vi "Retrieve and visualize_noDVR.vi"(11 "Field/Temperature":i32(slide) min=0 max=36 step=1) -> (1 "slowest":dbl format="%#_6p")   [LabVIEW 2020, in "Retrieve and Visualize.lvclass"]
uses:
  Retrieve and Visualize.lvclass
  typedefs/IV Setup--Cluster.ctl
  typedefs/Choose Intensity Data--enum.ctl
  <userlib>/LevyLab/LV-Data/LV-Data/Typedefs/File Type--enum.ctl
  typedefs/Choose XY Data--enum.ctl
  <userlib>/LevyLab/Graph Utilities/graph_utilities.lvclass
  <userlib>/LevyLab/Instrument Framework/SMOs/Configuration/Configuration.lvclass
  typedefs/INI--Cluster.ctl
  <vilib>/Utility/sysdir.llb/System Directory Type.ctl
  <userlib>/LevyLab/Graph Utilities/graph_utilities.lvclass/graph_utilities.ctl
  Retrieve and Visualize.lvclass/Retrieve and Visualize.ctl
  <userlib>/LevyLab/XY Utilities/subVIs/Subset (multiple).vi
  <userlib>/LevyLab/XY Utilities/subVIs/Sort (multiple).vi
  <userlib>/LevyLab/XY Utilities/subVIs/Decimate (multiple).vi
  <userlib>/LevyLab/XY Utilities/subVIs/Savitsky Golay Filter (multiple).vi
  <userlib>/LevyLab/XY Utilities/subVIs/Difference Quotient (multiple).vi
  <vilib>/Analysis/baseanly.llb/A x B.vi
  <vilib>/Analysis/baseanly.llb/A x Vector.vi
  <userlib>/LevyLab/XY Utilities/subVIs/Subset (single).vi
  <userlib>/LevyLab/XY Utilities/subVIs/Sort (single).vi
  <userlib>/LevyLab/XY Utilities/subVIs/Decimate (single).vi
  <userlib>/LevyLab/XY Utilities/subVIs/Savitsky Golay Filter (single).vi
  <userlib>/LevyLab/XY Utilities/subVIs/Difference Quotient (single).vi
  <vilib>/Analysis/2dsp.llb/Decimate (single shot).vi
  <vilib>/Analysis/2dsp.llb/Decimate (single shot, DBL).vi
  <vilib>/Analysis/3filter.llb/Savitzky-Golay Filter.vi
  <vilib>/Analysis/3filter.llb/Savitzky-Golay Filter (DBL).vi
  <userlib>/LevyLab/XY Utilities/Private/X Units.vi
  <userlib>/LevyLab/XY Utilities/Swap X and Y.vi
  <userlib>/LevyLab/XY Utilities/subVIs/Swap X and Y (single).vi
  <userlib>/LevyLab/XY Utilities/Private/DQ subVI.vi
  <userlib>/LevyLab/XY Utilities/Reverse.vi
  <userlib>/LevyLab/XY Utilities/subVIs/Reverse (single).vi
  <userlib>/LevyLab/XY Utilities/Divide.vi
  <userlib>/LevyLab/XY Utilities/subVIs/Divide float (single).vi
  <userlib>/LevyLab/XY Utilities/Add.vi
  <userlib>/LevyLab/XY Utilities/subVIs/Add XY (single).vi
  <userlib>/LevyLab/XY Utilities/Private/X Array Range to Index.vi
  <userlib>/LevyLab/Graph Utilities/Intensity Graph/Set Intensity Graph Cursor.vi
  <userlib>/LevyLab/Graph Utilities/Intensity Graph/Get Intensity Graph X Scale.vi
  <userlib>/LevyLab/Graph Utilities/Intensity Graph/Get Intensity Graph Value.vi
  <userlib>/LevyLab/Graph Utilities/Intensity Graph/Get Intensity Graph Y Scale.vi
  <userlib>/LevyLab/Graph Utilities/subVIs/Step Average.vi
  <userlib>/LevyLab/Graph Utilities/subVIs/Normalized Gaussian.vi
  <userlib>/LevyLab/Graph Utilities/XY Graph/Set XY Graph Value (array).vi
  <userlib>/LevyLab/Graph Utilities/Intensity Graph/Get Intensity Graph Y Label.vi
  <userlib>/LevyLab/Graph Utilities/XY Graph/Set XY Graph X Label.vi
  <userlib>/LevyLab/Graph Utilities/Intensity Graph/Get Intensity Graph Z Label.vi
  <userlib>/LevyLab/Graph Utilities/XY Graph/Set XY Graph Y Label.vi
  <userlib>/LevyLab/Graph Utilities/Intensity Graph/Get Intensity Graph X Label.vi
  <userlib>/_OpenG.lib/file/file.llb/File Exists - Scalar__ogtk.vi
  <userlib>/_OpenG.lib/array/array.llb/Sort Array__ogtk.vi
  <userlib>/_OpenG.lib/array/array.llb/Sort 1D Array (DBL)__ogtk.vi
  <userlib>/_OpenG.lib/array/array.llb/Reorder Array2__ogtk.vi
  <userlib>/_OpenG.lib/array/array.llb/Reorder 1D Array2 (DBL)__ogtk.vi
  <vilib>/Analysis/NI_AAL_SigProc.lvlib
  <userlib>/LevyLab/XY Utilities/xy_utilities.lvlib
  <userlib>/LevyLab/XY Utilities/subVIs/Interpolate (single).vi
  <userlib>/LevyLab/XY Utilities/Typedefs/Interpolation Configuration--cluster.ctl
  <userlib>/LevyLab/LV-Data/LV-Data.ITX/LV-Data.ITX.lvclass
  <userlib>/LevyLab/LV-Data/LV-Data/LV-Data.lvclass
panel:
  out "Status":string
  in  "Tab Control 2":enum32{"Sweep Control", "Visualize"}(tab)=enum."Visualize"
  out "Cursor Graph":cluster{dbl[], dbl[]}(graph)={[0.099856, 0.1204, 0.1401, 0.1599, 0.1798, 0.1998, 0.2198, 0.2398, 0.2598, 0.2798, 0.2998, 0.3199, 0.3398, 0.3598, 0.3798, 0.4, 0.4196, 0.4398, 0.4598, 0.4796, 0.5, 0.52, 0.5399, 0.5597, 0.5799, 0.5997, 0.62, 0.6398, 0.6601, 0.68, 0.6997, 0.7198, 0.7399, 0.7598, 0.78, 0.8002, 0.8201, 0.8401, 0.8597, 0.8797, 0.9, 0.9198, 0.9399, 0.96, 0.9798, 0.9802, 1.0002, 1.0202, 1.0404, 1.0602, 1.0807], [0.999930859375, 0.999930859375, 0.999930859375, 0.999930859375, 0.999930859375, 0.999930859375, 0.999930859375, 0.999930859375, 0.999930859375, 0.999930859375, 0.999930859375, 0.999930859375, 0.999930859375, 0.999930859375, 0.999930859375, 0.999930859375, 0.999930859375, 0.999930859375, 0.999930859375, 0.999930859375, 0.999930859375, 0.999930859375, 0.999930859375, 0.999930859375, 0.999930859375, 0.999930859375, 0.999930859375, 0.999930859375, 0.999930859375, 0.999930859375, 0.999930859375, 0.999930859375, 0.999930859375, 0.999930859375, 0.999930859375, 0.999930859375, 0.999930859375, 0.999930859375, 0.999930859375, 0.999930859375, 0.999930859375, 0.999930859375, 0.999930859375, 0.999930859375, 0.999930859375, 0.999930859375, 0.999930859375, 0.999930859375, 0.999930859375, 0.999930859375, 0.999930859375]}
  out "Fast":dbl=-2.603786046511628
  out "Slow":dbl=0.023622047244094446
  in  "decimating factor (1)":i32=1
  in  "averaging":bool
  in  "S-G side points (2T)":i32=10
  in  "S-G side points (4T)":i32=10
  in  "Subset Slider (%) A":cluster{dbl, dbl}(slide)={100.0, 0.0} scale=0.0..100.0 scale format="%#_6f"
  in  "Window [h]":dbl=10.0 min=2.0
  in  "Transconductance [h]":dbl=10.0 min=2.0
  in  "Visualize Button":bool
  in  "Open DAT Path":path=path "G:/.shortcut-targets-by-id/0B8-gGFa6hkR4XzJJMDlqZXVKRk0/ansom/Data/PPMS 3/SA40511C.20250205/000-processed/10-IV1TWire1nd2_Tsweep.000002.dat"
  in  "Macro: Visualize":string="Data Visualize: Read DAT File\nData Visualize: Initialize Graphs\nData Visualize: Initialize Cursor Graph\nData Visualize: Subset\nData Visualize: Testing\nData Visualize: SG Filter\nData Visualize: Calculate Derivative 2T\nData Visualize: Calculate Derivative 4T\nData Visualize: IV 4T IV 2T\n//Data Visualize: Calculate Transconductance\nData Visualize: Calculate Indices\nGraph: Initialize\nGraph: Set Y\nGraph: Set Labels\n//Data Visualize: Calculate Indices\n//Data Visualize: Choose Data 1\n//Data Visualize: Choose Data 2\n//Graph: Linecuts\n//UI: Choose Tab >> Intensity Graphs\nUI: Cursor Set >> Idle"
  in  "OK":bool
  in  "Tab Control":T1(tab)=enum."Intensity Graphs"
  out "Comments":string="      #Vslow/#Vfast/# of IV curves/BT offset/#discarded IV curves/Manual offset:\n /1/51/1/0/0/0    \n#of fields: 1    \nField period 1 \nDecimate point 1.000000 \nScan names \nT (K)\nB (T)\nappliedField \n Device: \r  Device Name: SA40511C.20250205\r  Computer: PPMS3DAQ\r  User: Ranjani\r  Instrument: PPMS 3\r  Description: |\r    LAO/KTO 3wire Nernst\r\rExperiment: \r  Time: 2025-02-08T22:02:51\r  Description: |\r    T = 100mK to 980mK, 20mK step,10K/min \r    Wait(temperature)\r    B= 1T\r    \r    I1 and 2+= 0 to -50m to 50m to 0V, 30s\r    wait, 2s\r    I+/- = 2/5\r    V+/- = 1/26\r    I2+/- = 3/4\r    Wire 3\r    I3+/- = 0 mV\r\rSweep: \r- Loop1: [Temperature, 1.080000]\r- Loop2: [OFF, -14.000000]\r- Loop3: [OFF, 0.000000]\r- Loop4: [OFF, 0.000000]\r\rWiring: \r- Electrode 1: Lockin 1, V1+\r- Electrode 2: Lockin 2, I+\r- Electrode 3: Lockin 3, I2+\r- Electrode 4: Lockin 4, I2-\r- Electrode 5: Lockin 5, I-\r- Electrode 26: Lockin 6, V1-\r- Electrode 27: Lockin 7, I3+\r- Electrode 28: Lockin 8, I3+\r\rLockin: \r  AO: \r  - AO 1: amp = 0.000 mV, DC = 0.000 mV, f = 13.00 Hz, phi = 0.00°, Sine\r  - AO 2: amp = 0.000 mV, DC = 0.001 mV, f = 13.00 Hz, phi = 0.00°, Sine\r  - AO 3: amp = 0.000 mV, DC = 0.001 mV, f = 13.00 Hz, phi = 0.00°, Sine\r  - AO 4: amp = 0.000 mV, DC = 0.000 mV, f = 13.00 Hz, phi = 0.00°, Sine\r  - AO 5: amp = 0.000 mV, DC = 0.000 mV, f = 13.00 Hz, phi = 0.00°, Sine\r  - AO 6: amp = 0.000 mV, DC = 0.000 mV, f = 13.00 Hz, phi = 0.00°, Sine\r  - AO 7: amp = 0.000 mV, DC = 0.000 mV, f = 13.00 Hz, phi = 0.00°, Sine\r  - AO 8: amp = 0.000 mV, DC = 0.000 mV, f = 13.00 Hz, phi = 0.00°, Sine\r  REF: \r  - Lockin 1: f = 13.00 Hz, phi = 0.00°, TC = 0.10 s, order = 2 \r  - Lockin 2: f = 26.00 Hz, phi = 0.00°, TC = 0.10 s, order = 2 \r  Sampling: \r  - Fs: 13000.000000\r  - N: 1000\r"
  in  "index":T2={"I-(A)"="AO2", "I+(A)"="AI5", "V4T+"="AI1", "V4T-"="AI6", "UG"="AO1", "DG"="AO1", "LG"="AO6", "B"="Magnet", "Temperature"="Temperature", "Vfast"="Temperature", "Vslow"="Magnet"}
  in  "Check Files Button":bool
  in  "Generate Button":bool
  in  "Additional comments":string
  in  "Field Period":i32=1
  in  "# of fields/Temperatures":i32=1
  in  "Path":path=path "G:/.shortcut-targets-by-id/0B8-gGFa6hkR4XzJJMDlqZXVKRk0/ansom/Data/PPMS 3/SA40511C.20250205/10-IV1TWire1nd2_Tsweep"
  in  "DAT folder":path=path "G:/.shortcut-targets-by-id/0B8-gGFa6hkR4XzJJMDlqZXVKRk0/ansom/Data/PPMS 3/SA40511C.20250205/000-processed"
  in  "IV setup":T3={"# Vslow"=1, "# Vfast"=51, "#IV Curves at each gate"=1, "B/T offset"=0, "Discard first # curves"=0, "Manual offset"=0}
  in  "Scan names":string[](array[string])=["T (K)", "B (T)", "appliedField"]
  in  "Portion of data (%)":cluster{dbl, dbl}(slide)={100.0, 0.0} scale=0.0..100.0
  in  "Decimate point":dbl=1.0 format="%#_1f"
  in  "Extract paramaters from comments?":bool
  in  "T/B third axis":bool
  in  "File Type":T4=enum."TDMS"
  in  "Export ITX Path":path
  in  "Export ITX":bool
  in  "Export What?":T5(ring)
  in  "Export ITX Name":string
  out "IV 4T":cluster{dbl[], dbl[]}[](graph)
  out "dI/dV (G)":cluster{dbl[], dbl[]}[](graph)
  out "dI/dV (G) 2T":cluster{dbl[], dbl[]}[](graph)
  out "IV 2T":cluster{dbl[], dbl[]}[](graph)
  out "dV/dI (R)":cluster{dbl[], dbl[]}[](graph)
  out "dV/dI (R) 2T":cluster{dbl[], dbl[]}[](graph)
  in  "XY Data":T6
  in  "fake point 1":dbl format="%#_6p"
  in  "Log scale? 1":bool
  in  "e^2/h? 1":bool
  in  "e^2/h? 2":bool
  in  "Log scale? 2":bool
  in  "fake point 2":dbl=-2.0 format="%#_6p"
  in  "Intensity 1":T7=enum."R-4T"
  out "Intensity Graph 1":dbl[][](graph)
  out "Intensity Graph 2":dbl[][](graph)
  out "H Cut 1":cluster{dbl[], dbl[]}[](graph)
  out "V Cut 1":cluster{dbl[], dbl[]}[](graph)=[{[0.099856, 0.11947288, 0.13908976, 0.15870664, 0.17832352, 0.19794040000000002, 0.21755728, 0.23717416, 0.25679103999999997, 0.27640792000000003, 0.2960248, 0.31564168000000004, 0.33525856, 0.35487544, 0.37449232, 0.3941092, 0.41372608, 0.43334296, 0.45295984, 0.47257672, 0.4921936, 0.5118104800000001, 0.53142736, 0.55104424, 0.57066112, 0.590278, 0.6098948799999999, 0.62951176, 0.64912864, 0.6687455200000001, 0.6883623999999999, 0.70797928, 0.72759616, 0.7472130399999999, 0.7668299199999999, 0.7864468, 0.8060636800000001, 0.8256805599999999, 0.84529744, 0.86491432, 0.8845312000000001, 0.9041480799999999, 0.92376496, 0.94338184, 0.9629987200000001, 0.9826155999999999, 1.00223248, 1.02184936, 1.0414662399999999, 1.06108312, 1.0807], [nan, nan, nan, nan, nan, nan, nan, nan, nan, nan, nan, nan, nan, nan, nan, nan, nan, nan, nan, nan, nan, nan, nan, nan, nan, nan, nan, nan, nan, nan, nan, nan, nan, nan, nan, nan, nan, nan, nan, nan, nan, nan, nan, nan, nan, nan, nan, nan, nan, nan, nan]}]
  out "H Cut 2":cluster{dbl[], dbl[]}[](graph)
  out "V Cut 2":cluster{dbl[], dbl[]}[](graph)=[{[0.099856, 0.11947288, 0.13908976, 0.15870664, 0.17832352, 0.19794040000000002, 0.21755728, 0.23717416, 0.25679103999999997, 0.27640792000000003, 0.2960248, 0.31564168000000004, 0.33525856, 0.35487544, 0.37449232, 0.3941092, 0.41372608, 0.43334296, 0.45295984, 0.47257672, 0.4921936, 0.5118104800000001, 0.53142736, 0.55104424, 0.57066112, 0.590278, 0.6098948799999999, 0.62951176, 0.64912864, 0.6687455200000001, 0.6883623999999999, 0.70797928, 0.72759616, 0.7472130399999999, 0.7668299199999999, 0.7864468, 0.8060636800000001, 0.8256805599999999, 0.84529744, 0.86491432, 0.8845312000000001, 0.9041480799999999, 0.92376496, 0.94338184, 0.9629987200000001, 0.9826155999999999, 1.00223248, 1.02184936, 1.0414662399999999, 1.06108312, 1.0807], [3.3762685773770134e-05, 2.3916778489875587e-05, 2.654588549110859e-05, 3.7526761290691605e-05, 3.2301327892542505e-05, 2.6454434035762424e-05, 2.652299633224866e-05, 3.230184057865135e-05, 1.959244546016357e-05, 2.584103725701611e-05, 3.445648987553342e-05, 1.7963722001670446e-05, 1.4959654834668283e-05, 2.488740425029002e-05, 2.6029819241313776e-05, 2.0114406725304238e-05, 2.1938239917722983e-05, 2.3924326114769558e-05, 1.688456387309341e-05, 1.2689595493509836e-05, 2.1639531028779784e-05, 1.0262319510907414e-05, -2.2562712513605623e-06, 6.229663764846753e-06, 6.290560504043035e-06, -4.464216464504397e-06, -9.063974731389205e-06, 4.423251858920318e-06, -9.326548951846347e-06, -1.0215397278681526e-05, -9.304831257511187e-06, -8.915859738611292e-06, -1.9912084696571762e-05, -9.449798911587456e-06, -1.145229397349045e-05, -1.7712755942352026e-05, -2.02944113979962e-05, -1.313296945631493e-05, -2.420582028533799e-05, -2.348366665214838e-05, -1.8166676626836458e-05, -2.5173787476635757e-05, -3.2642280402476225e-05, -1.8777899023935893e-05, -2.788070158268089e-05, -7.192029457748351e-06, -1.8816023944703815e-05, -1.6190991731435217e-05, -1.1918852338953221e-05, -1.8801482914666336e-05, -2.1966004211086435e-05]}]
  in  "Intensity 2":T7
  in  "X Offset 1":dbl format="%#_6p"
  in  "X Offset 2":dbl format="%#_6p"
  out "x3D Graph 11":dbl[][](graph)
  out "x3D Graph 10":dbl[][](graph)
  out "x3D Graph 9":dbl[][](graph)
  out "x3D Transconductance 2":dbl[][](graph)
  in  "Intensity 3D":T7=enum."G-4T"
  out "bottom loop":dbl[](graph)
  out "xalpha top loop":dbl[](graph)
  out "xalpha Top loop Intensity Graph":dbl[][](graph)
  out "xalpha Vsd vs Vsg":cluster{dbl[], dbl[]}(graph)
  in  "xalpha threshold 2":dbl format="%0.2f"
  in  "xalpha width 2":i32=3 min=3
  out "xalpha Y line cut 9":cluster{dbl[], dbl[]}[](graph)
  out "xalpha Vsg?":dbl[](array[numeric])
  out "xalpha vertical peak diff":dbl[](array[numeric])
  in  "xalpha threshold":dbl format="%0.2f"
  in  "xalpha width":i32=3 min=3
  in  "xalpha derivative bin size":dbl=10.0
  in  "Diff Interval":dbl=12.0
  in  "derivative bin size 2":dbl
  in  "derivative bin size 1":dbl
  in  "SG Filter?":bool=TRUE
  # "Input"
  # "Process Parameters"
  # "obsolete?"
  # "Vfast"
  # "Vslow"
  # "Vslowest"
  # "Output"
  # "#todo: add button to automatically populate output and filename fields"
  # "Used??"
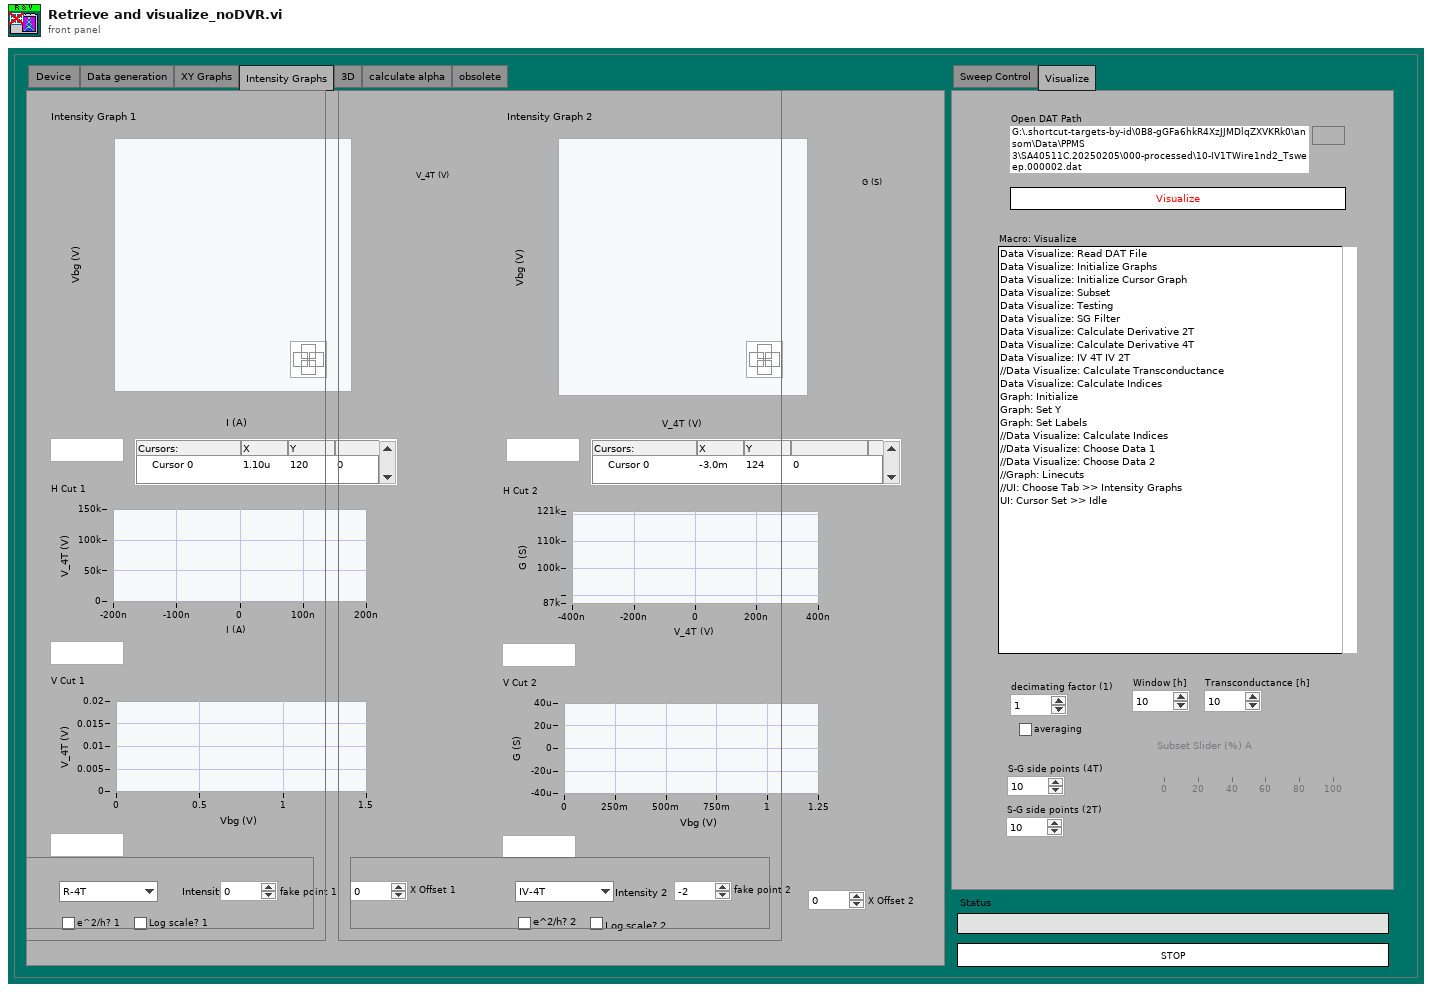
[diagram p1: front panel]
types:
  T1 = enum32{"Device ", "Data generation", "XY Graphs", "Intensity Graphs", "3D", "calculate alpha", "obsolete"}
  T2 = cluster{"I-(A)":string, "I+(A)":string, "V4T+":string, "V4T-":string, "UG":string, "DG":string, "LG":string, "B":string, "Temperature":string, "Vfast":string, "Vslow":string}
  T3 = typedef "Retrieve and Visualize.lvclass/IV Setup--Cluster.ctl" = cluster{"# Vslow":i32, "# Vfast":i32, "#IV Curves at each gate":i32, "B/T offset":i32, "Discard first # curves":i32, "Manual offset":i32}
  T4 = typedef "LV-Data.lvclass/File Type--enum.ctl" = enum16{"DAT", "ITX", "TDMS", "VI"}
  T5 = enum16{"Intensity 1", "H Cut 1", "V Cut 1", "Intensity 2", "H Cut 2", "V Cut 2"}
  T6 = typedef "Retrieve and Visualize.lvclass/Choose XY Data--enum.ctl" = enum16{"Vary Vfast", "Vary Vslow", "Vary Fields"}
  T7 = typedef "Retrieve and Visualize.lvclass/Choose Intensity Data--enum.ctl" = enum16{"IV-4T", "IV-2T", "R-4T", "G-4T", "R-2T", "G-2T", "dGdVsg-4T", "dGdVsg-2T"}
  T8 = enum32{"Device ", "Data generation", "Vary Vfast", "Vary Vslow", "Vary Fields", "Intensity Graphs", "3D (disabled)", "calculate alpha (disabled)"}
  T9 = cluster{"IV-4T":refnum<data-value>, "G-2T":refnum<data-value>, "R-2T":refnum<data-value>, "G-4T":refnum<data-value>, "R-4T":refnum<data-value>, "IV-2T":refnum<data-value>, "Vfast":dbl[][], "Vslow":dbl[], "Vslowest":dbl[], "Scan Names":string[]}
  T10 = typedef "xy_utilities.lvlib/Interpolation Configuration--cluster.ctl" = cluster{"X Low":dbl, "X High":dbl, "X Step":dbl, "Fake Point":dbl}
  T11 = typedef "LVOffsetAndMultiplierTypeDef.ctl" = cluster{"Offset":dbl, "Multiplier":dbl}
  T12 = enum32{"Invalid", "Standard", "Closed", "Hidden", "Minimized", "Maximized"}
  T13 = enum32{"invalid app kind", "Development System", "Run Time System", "Student Edition", "Embedded LabVIEW", "Evaluation", "Custom"}
  T14 = typedef "Retrieve and Visualize.lvclass/INI--Cluster.ctl" = cluster{"Open DAT Path":path, "Export ITX Path":path, "Export ITX Name":string, "Intensity 1":T7, "X Offset 1":dbl, "derivative bin size 1":dbl, "e^2/h? 1":bool, "Log scale? 1":bool, "fake point 1":dbl, "Intensity 2":T7, "X Offset 2":dbl, "derivative bin size 2":dbl, "e^2/h? 2":bool, "Log scale? 2":bool, "fake point 2":dbl}
  T15 = cluster{"Core":cluster{"Current VI Reference":refnum<vi>, "Close Panel on Exit?":bool}, "R&V":refnum<class "Retrieve and Visualize.lvclass">, "Configuration":refnum<class "Configuration.lvclass">, "INI":T14, "3D":cluster{"IV-4T":cluster{dbl[], dbl[]}[][][], "IV-2T":cluster{dbl[], dbl[]}[][][], "G-4T":cluster{dbl[], dbl[]}[][][], "R-4T":cluster{dbl[], dbl[]}[][][], "G-2T":cluster{dbl[], dbl[]}[][][], "R-2T":cluster{dbl[], dbl[]}[][][], "dG-4T":cluster{dbl[], dbl[]}[][][], "Differential Mode":cluster{dbl[], dbl[]}[][][], "Common Mode":cluster{dbl[], dbl[]}[][][]}, "Graph":cluster{"Intensity 1":refnum<class "graph_utilities.lvclass">, "V 1":refnum<class "graph_utilities.lvclass">, "H 1":refnum<class "graph_utilities.lvclass">, "Intensity 2":refnum<class "graph_utilities.lvclass">, "V 2":refnum<class "graph_utilities.lvclass">, "H 2":refnum<class "graph_utilities.lvclass">}, "Vfast":dbl[][], "Vslow":dbl[], "Vslowest":dbl[], "Scan Names":string[], "Vfast Slice":dbl[], "Vslow Slice":dbl[], "Page":i32, "Row":i32, "Column":i32, "Row []":i32[], "Column []":i32[], "V2T":dbl[]}
  T16 = cluster{"Intensity 1":refnum<class "graph_utilities.lvclass">, "V 1":refnum<class "graph_utilities.lvclass">, "H 1":refnum<class "graph_utilities.lvclass">, "Intensity 2":refnum<class "graph_utilities.lvclass">, "V 2":refnum<class "graph_utilities.lvclass">, "H 2":refnum<class "graph_utilities.lvclass">}
  T17 = cluster{"IV-4T":cluster{dbl[], dbl[]}[][][], "IV-2T":cluster{dbl[], dbl[]}[][][], "G-4T":cluster{dbl[], dbl[]}[][][], "R-4T":cluster{dbl[], dbl[]}[][][], "G-2T":cluster{dbl[], dbl[]}[][][], "R-2T":cluster{dbl[], dbl[]}[][][], "dG-4T":cluster{dbl[], dbl[]}[][][], "Differential Mode":cluster{dbl[], dbl[]}[][][], "Common Mode":cluster{dbl[], dbl[]}[][][]}
  T18 = cluster{"Current VI Reference":refnum<vi>, "Close Panel on Exit?":bool}
  T19 = typedef "System Directory Type.ctl" = i32
  T20 = typedef "LVPointDoubleTypeDef.ctl" = cluster{"X":dbl, "Y":dbl}
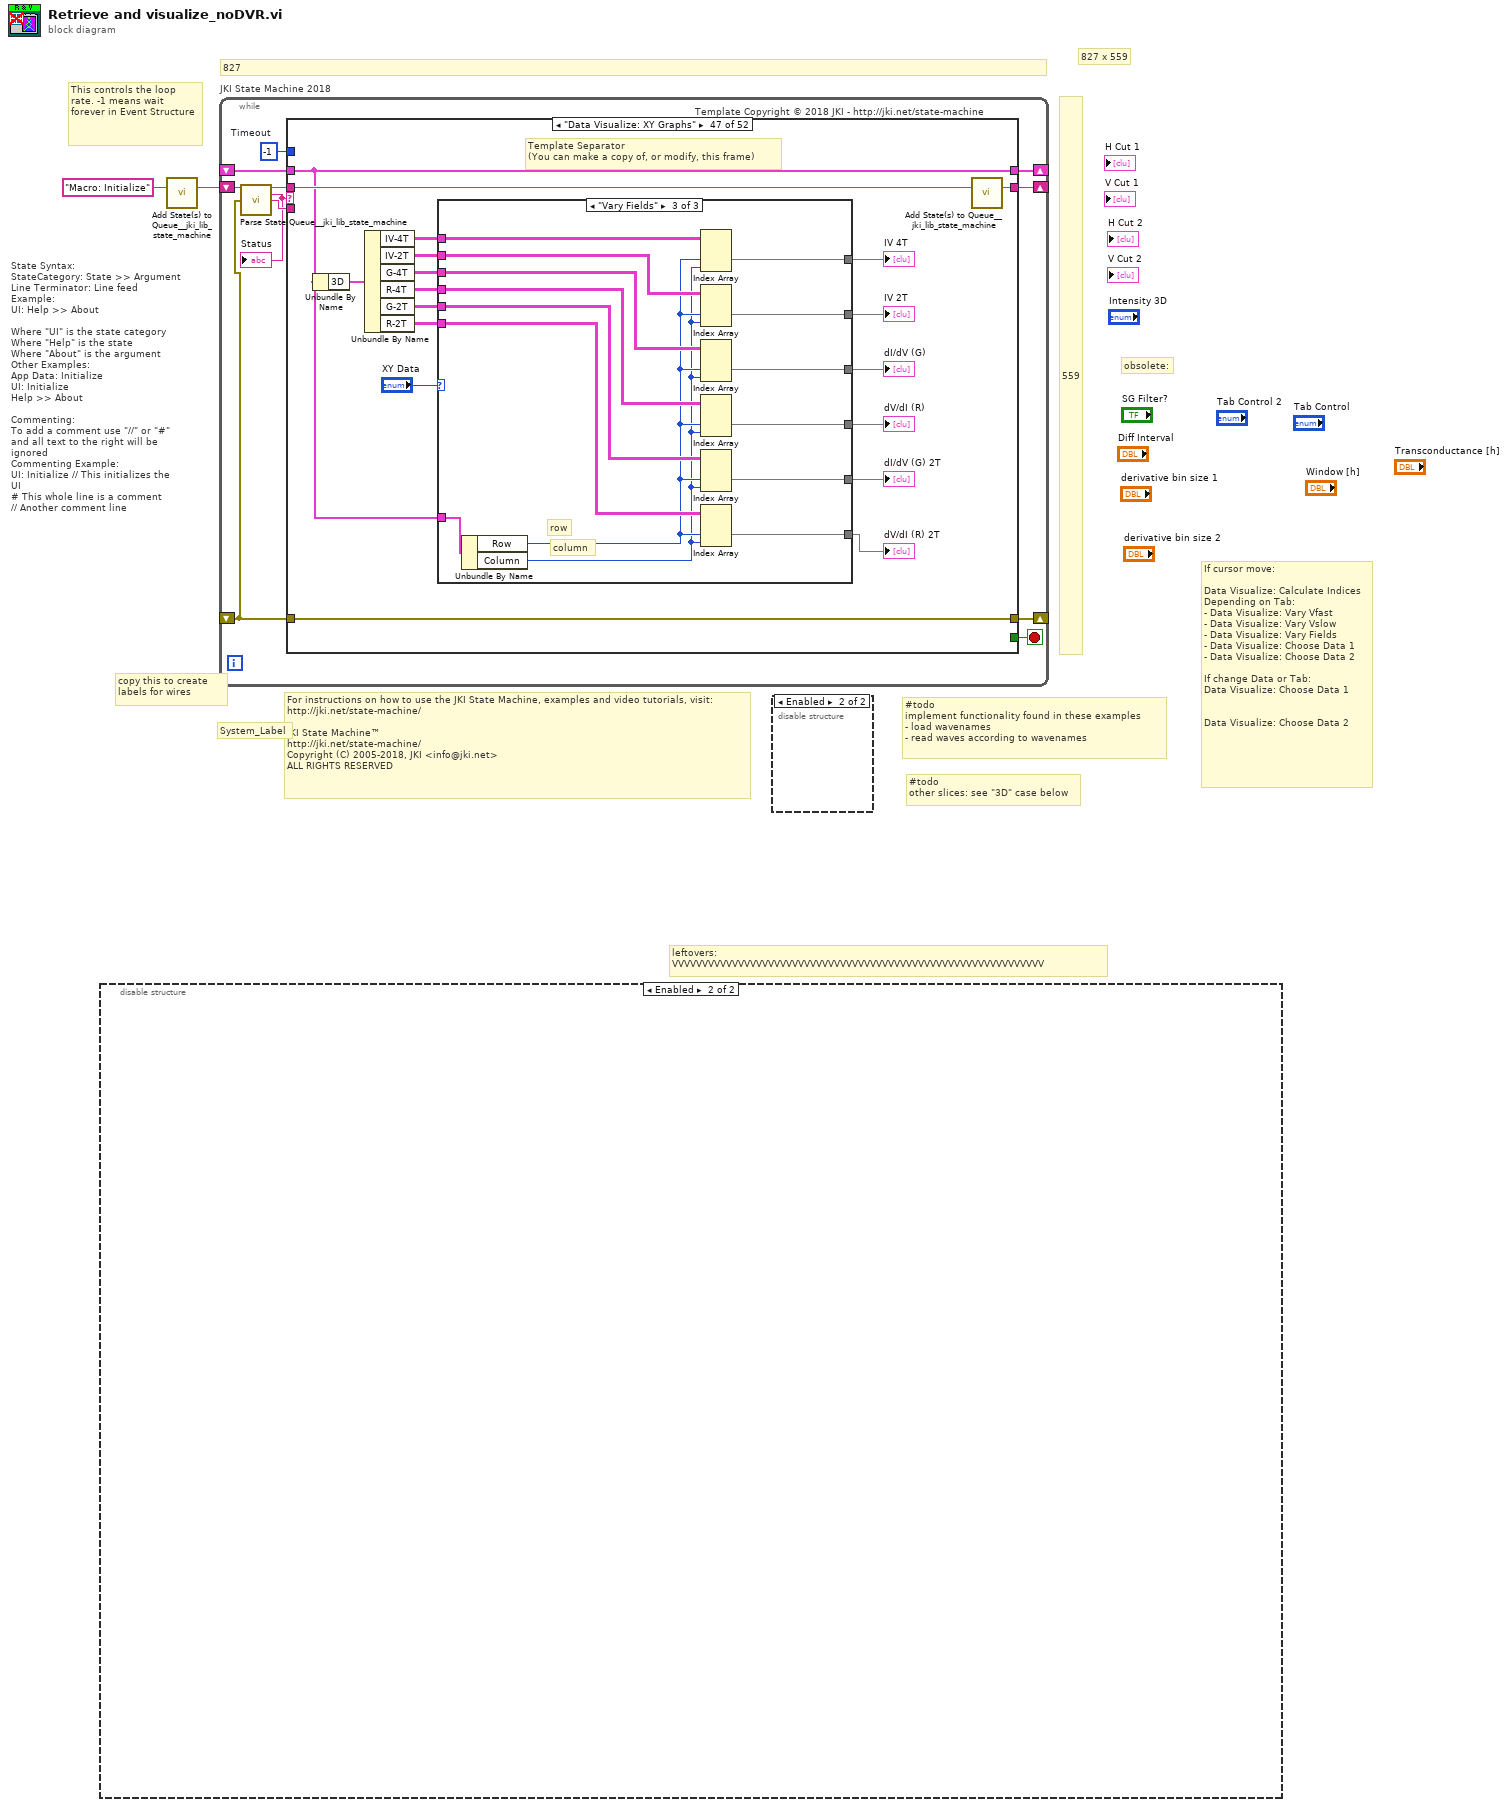
[diagram p0: block diagram]
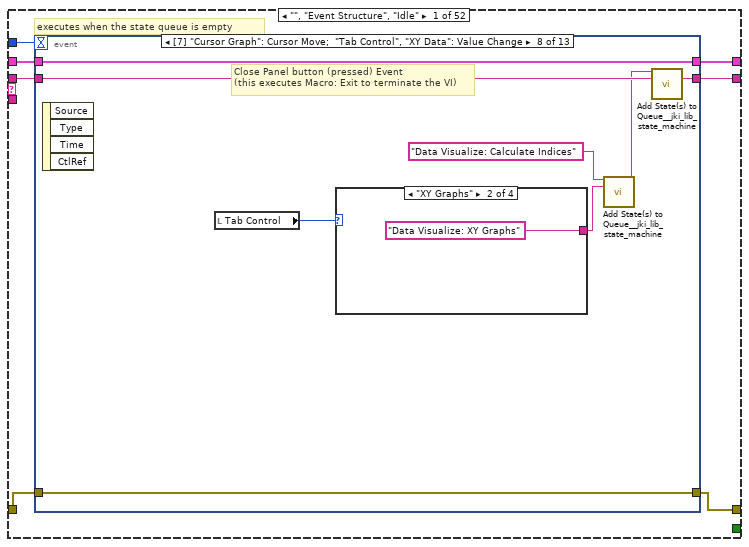
[diagram p2: hidden frame]
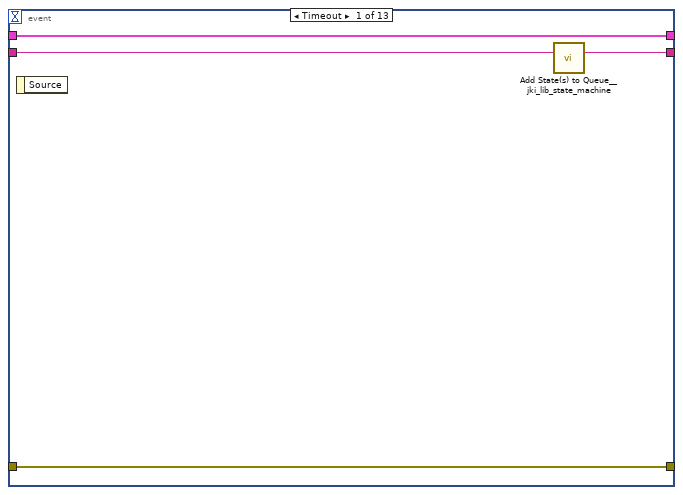
[diagram p3: hidden frame]
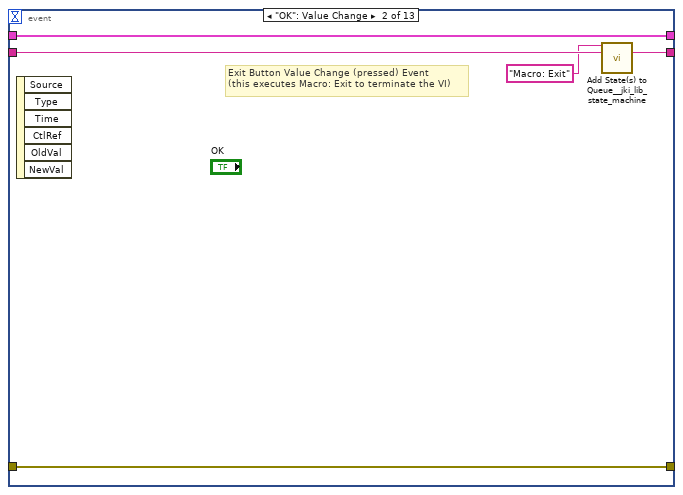
[diagram p4: hidden frame]
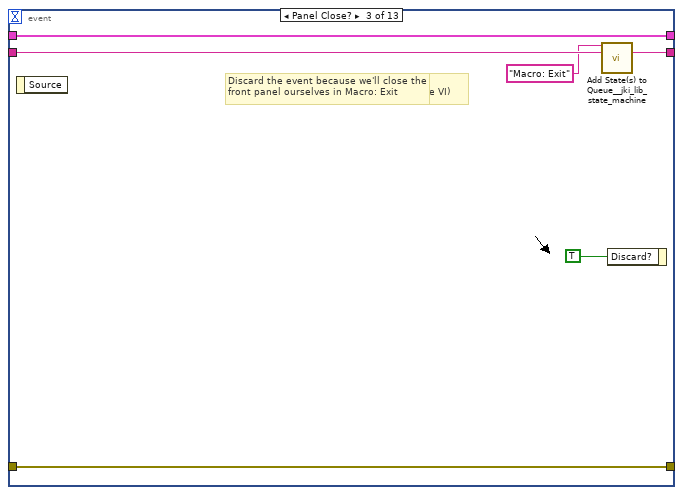
[diagram p5: hidden frame]
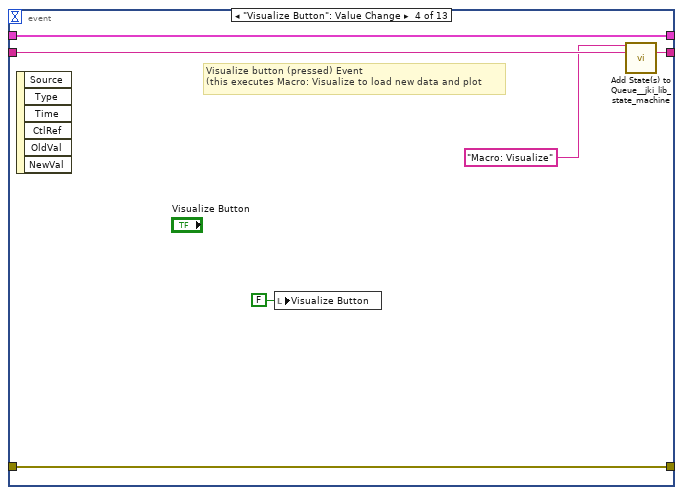
[diagram p6: hidden frame]
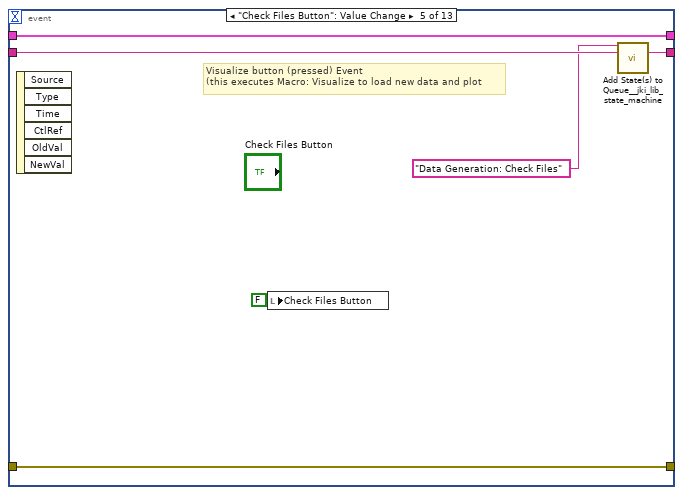
[diagram p7: hidden frame]
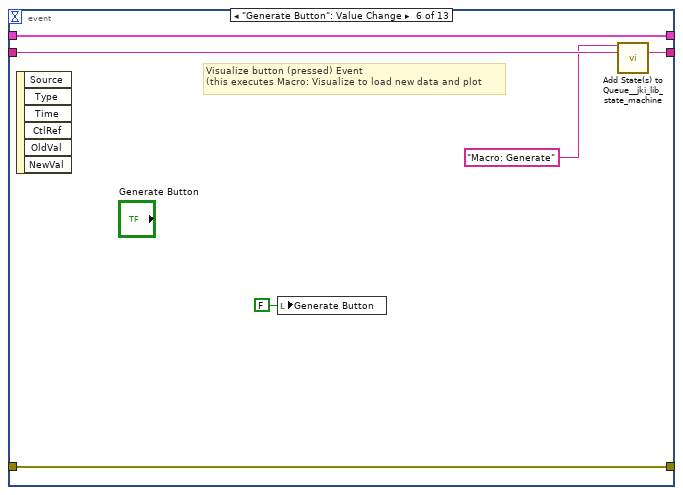
[diagram p8: hidden frame]
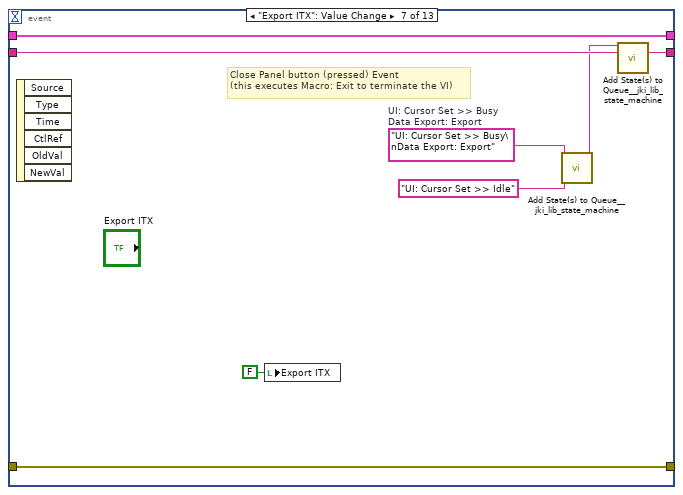
[diagram p9: hidden frame]
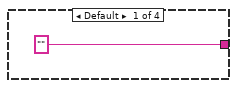
[diagram p10: hidden frame]
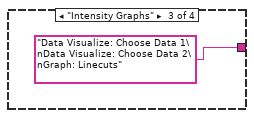
[diagram p11: hidden frame]
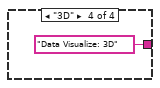
[diagram p12: hidden frame]
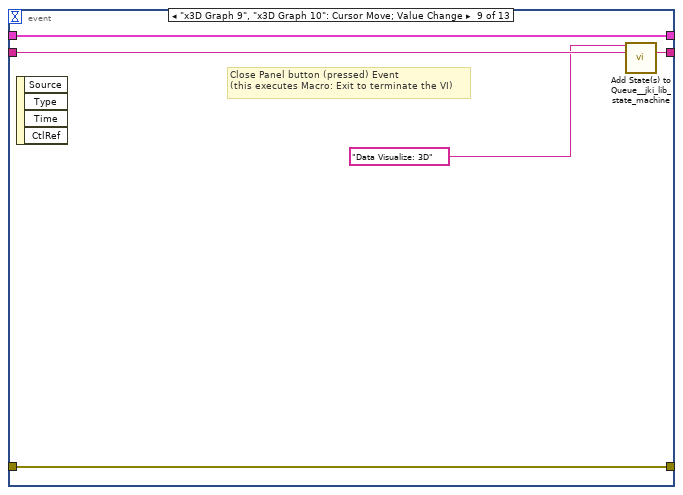
[diagram p13: hidden frame]
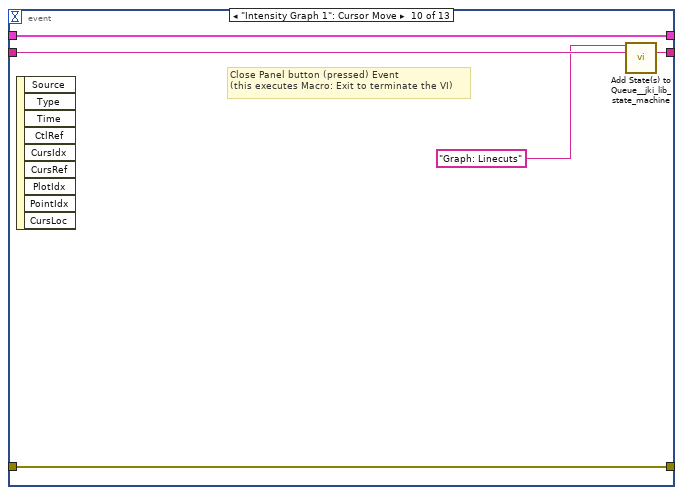
[diagram p14: hidden frame]
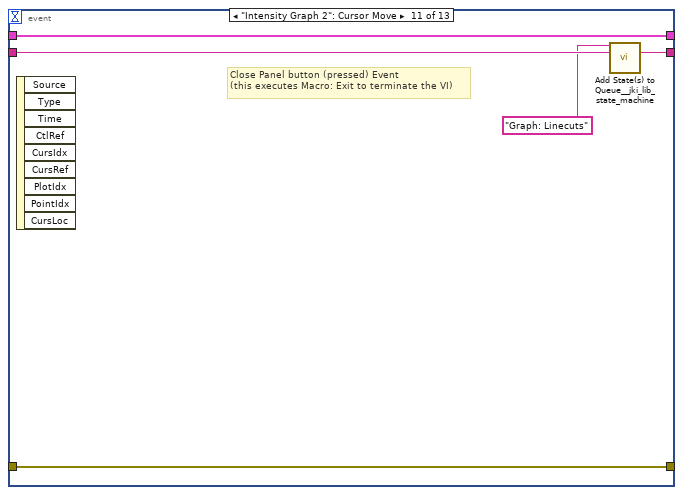
[diagram p15: hidden frame]
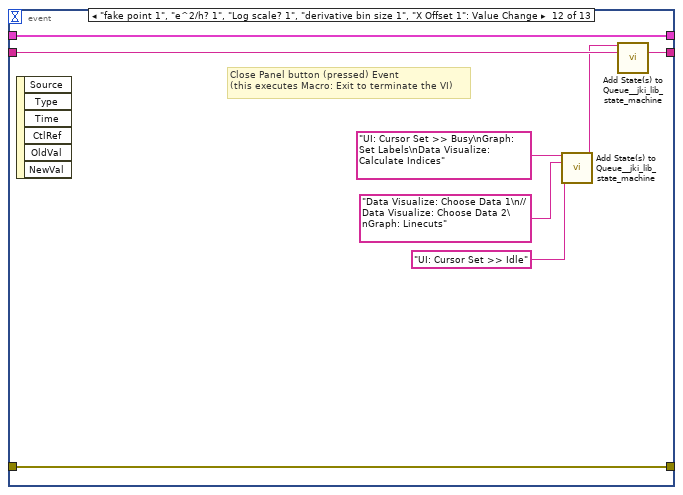
[diagram p16: hidden frame]
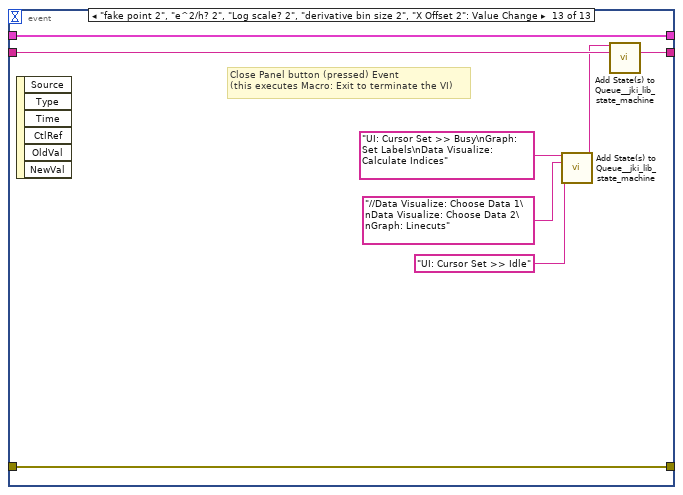
[diagram p17: hidden frame]
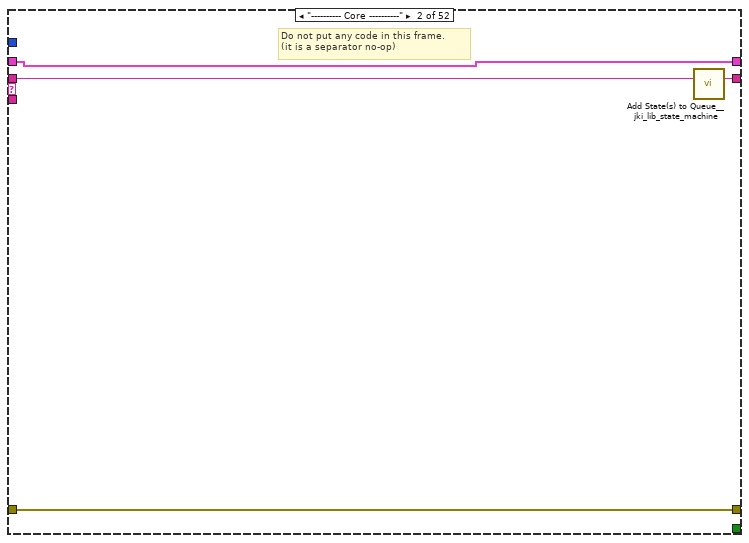
[diagram p18: hidden frame]
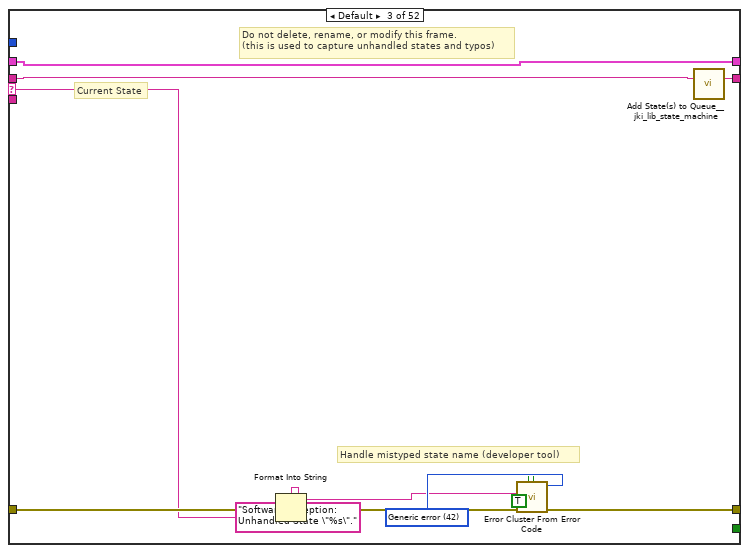
[diagram p19: hidden frame]
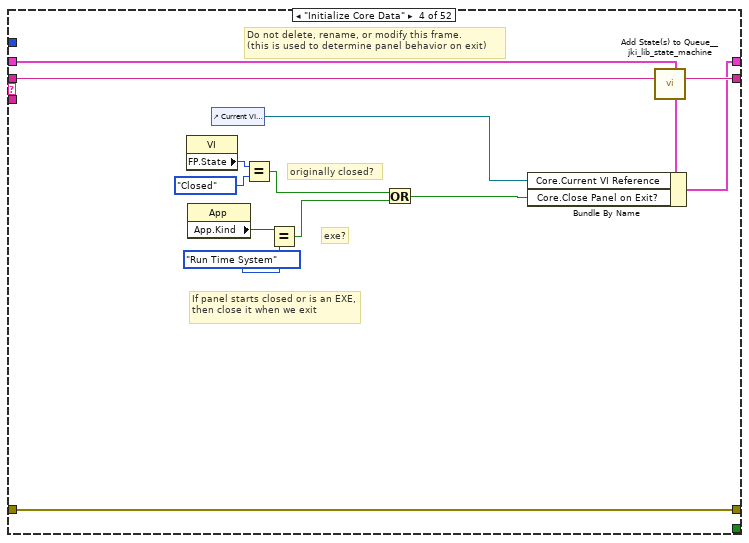
[diagram p20: hidden frame]
diagram:
  # "827"
  # "559"
  # "827 x 559"
  # "#todo\nother slices: see \"3D\" case below"
  # "#todo\nimplement functionality found in these examples\n- load wavenames\n- read waves according to wavenames"
  # "obsolete:"
  # "If cursor move:\n\nData Visualize: Calculate Indices\nDepending on Tab:\n- Data Visualize: Vary Vfast\n- Data Visualize: Vary Vslow\n- Data Visualize: Vary Fields\n- Data Visualize: Choose Data 1\n- Data Visualize: Choose Data 2\n\nIf change Data or Tab:\nData Visualize: Choose Data 1\n\n\nData Visualize: Choose Data 2"
  # "leftovers:\nVVVVVVVVVVVVVVVVVVVVVVVVVVVVVVVVVVVVVVVVVVVVVVVVVVVVVVVVVVVVVV"
  # "For instructions on how to use the JKI State Machine, examples and video tutorials, visit:\nhttp://jki.net/state-machine/\n\nJKI State Machine™\nhttp://jki.net/state-machine/\nCopyright (C) 2005-2018, JKI <info@jki.net>\nALL RIGHTS RESERVED"
  # "State Syntax:\nStateCategory: State >> Argument\nLine Terminator: Line feed\nExample:\nUI: Help >> About\n\nWhere \"UI\" is the state category\nWhere \"Help\" is the state\nWhere \"About\" is the argument\nOther Examples:\nApp Data: Initialize\nUI: Initialize\nHelp >> About\n\nCommenting:\nTo add a comment use \"//\" or \"#\" and all text to the right will be ignored\nCommenting Example:\nUI: Initialize // This initializes the UI\n# This whole line is a comment\n// Another comment line"
  # "copy this to create labels for wires"
  # "This controls the loop rate. -1 means wait forever in Event Structure"
  # "System_Label"
  n1 = disable-structure shown="Enabled" {
    frame Disabled {
      # "column"
      # "Y Vfast slice"
      # "Y Vslow slice"
      # "Y scale for \nSlice at constant B"
      # "row"
      # "col []"
      # "row []"
      # "page"
      # "Vslowest"
      # "Vslow"
      # "Vfast"
      n2 = for {
        tunnel: _ -> [w17] mode=indexing
        # "determine automatically"
        n3 = call-poly <userlib>:"Interpolate.vi"("Configure"=T10 {"X Low"=0.05, "X High"=0.5, "X Step"=0.01, "Fake Point"=0.05}, "XY-data"=w17) -> ("Interpolated XY-data out"=w16:cluster{"X-array":dbl[], "Y-array":dbl[]})  [unwired: 8 in, 1 out]
        n4 = Unbundle(w16) -> ()  [unwired: 2 out]
      }
      n5 = case shown="\"calculate alpha (disabled)\"" T8."Device " ("Tab Control") {
        tunnel: 0 ("Field/Temperature") -> [w23 _ _]
        tunnel: 0 ("Row") -> [w24 w41 _]
        tunnel: dbl[][] [] ("Vfast") -> [_ w39 _]
        tunnel: dbl[] [] ("Vslow") -> [_ w40 _]
        tunnel: dbl[] [] ("Vslowest") -> [_ _ _]
        tunnel: i32[] [] ("Row Array") -> [w22 _ _]
        tunnel: i32[] [] ("Column Array") -> [w21 _ _]
        tunnel: T9 {"IV-4T"=refnum, "G-2T"=refnum, "R-2T"=refnum, "G-4T"=refnum, "R-4T"=refnum, "IV-2T"=refnum, "Vfast"=[], "Vslow"=[], "Vslowest"=[], "Scan Names"=[]} -> [w18 w38 _]
        tunnel: dbl[] [] ("Vfast") -> [w19 w36 _]
        tunnel: dbl[] [] -> [_ _ _]
        tunnel: 0 ("Column") -> [_ _ _]
        frame "Intensity Graphs" {
          n6 = Unbundle By Name(w18) -> ("G-4T"=w20:refnum<data-value>)
          n7 = in-place {
            in-place-border: w24 -> [_]
            in-place-border: w23 -> [w28]
            in-place-border: w22 -> [w27]
            in-place-border: w21 -> [w26]
            in-place-border: w19 -> [_]
            # "page"
            # "3D array"
            # "row[]"
            # "col[]"
            # "Slice along Constant Vsg"
            n8 = in-place-dvr #1(w20) -> (w25:cluster{dbl[], dbl[]}[][][])  [unwired: 1 out]
            n9 = for {
              tunnel: w25 -> [w35]
              tunnel: w28 -> [w34]
              tunnel: w27 -> [w31] mode=indexing
              tunnel: w26 -> [w32] mode=indexing
              tunnel: [w33] -> _ mode=indexing
              n10 = Index Array(array=w35, index (dim 0)=w34, index (dim 1)=w31, index (dim 2)=w32) -> (element=w30:cluster{dbl[], dbl[]})
              n11 = call-poly <userlib>:"Interpolate.vi"("XY-data"=w30) -> ("Interpolated XY-data out"=w29:cluster{"X-array":dbl[], "Y-array":dbl[]})  [unwired: 9 in, 1 out]
              n12 = Unbundle(w29) -> ("Y-array"=w33:dbl[])  [unwired: 1 out]
            }
            n13 = in-place-dvr #1(w25) -> ()  [unwired: 2 out]
          }
        }
        frame "3D (disabled)" {
          n14 = Unbundle By Name(w38) -> ("G-4T"=w37:refnum<data-value>)
          n15 = in-place {
            in-place-border: w41 -> [_]
            in-place-border: w40 -> [_]
            in-place-border: w39 -> [_]
            in-place-border: w36 -> [_]
            n16 = in-place-dvr #2(w37) -> (w44:cluster{dbl[], dbl[]}[][][])  [unwired: 1 out]
            n17 = call "Derivative (2D).vi"("Window [h] (2)"="xalpha derivative bin size") -> ("Transconductance"=→"x3D Transconductance 2":dbl[][])  [unwired: 8 in, 2 out]
            n18 = property on="x3D Transconductance 2" class="IntGraph (strict)" props=["XScale", "Ofst&Mult", "YScale", "Ofst&Mult"]() -> ("YScale.Ofst&Mult"=w42:T11)  [unwired: 3 in, 2 out]
            n19 = in-place-dvr #2(w44) -> ()  [unwired: 2 out]
          }
        }
        frame "calculate alpha (disabled)" {
          n20 = disable-structure shown="Disabled" {
            frame Disabled {
              # "???????????????????????????????????????????????????????????????????????????????????????"
              # "4D data"
              # "Trans"
              # "B"
              # "current/Vsd"
              # "Vsg"
              n21 = Unbundle() -> (w61:T11, "Offset"=w52, "Multiplier"=w51)
              n22 = for {
                tunnel: [w95] -> w62 mode=indexing
                tunnel: [w104] -> w48 mode=indexing
                tunnel: w52 -> [w115]
                tunnel: w51 -> [w114]
                shift-right: [w111] -> w55
                shift-left: dbl[] [] -> [w109]
                tunnel: [w108] -> w49 mode=indexing
                tunnel: [w105] -> w59
                tunnel: [w96] -> w54 mode=indexing
                i -> [w113]
                n23 = Multiply(x=w114, y=w113) -> (x*y=w112:i32)
                n24 = Add(x=w115, y=w112) -> (x+y=w110:i32)
                n25 = call <vilib>:"Peak Detector.vi"("width"="xalpha width", "threshold"="xalpha threshold", "X"=w95) -> ("Locations"=w101:dbl[])  [unwired: 4 in, 4 out]
                n26 = Unbundle(w105) -> ("Offset"=w102, "Multiplier"=w103)
                n27 = Build Array (concatenate)(w109, w110) -> (w111:dbl[])
                n28 = Multiply(x=w101, y=w103) -> (x*y=w106:dbl[])
                n29 = Index Array(array=w101, index #1=0 ("index"), index #2=1 ("index")) -> (element #1=w108:dbl, element #2=w107:dbl)
                n30 = Add(x=w106, y=w102) -> (x+y=w100:dbl[])
                n31 = Subtract(x=w107, y=w108) -> (x-y=w104:dbl)
                n32 = Wait (ms)(milliseconds to wait=u32 10) -> ()  [unwired: 1 out]
                n33 = Index Array(array=w100, index #1=0 ("index"), index #2=1 ("index")) -> (element #1=w97:dbl, element #2=w98:dbl)
                n34 = Subtract(x=w98, y=w97) -> (x-y=w96:dbl)
                "bottom loop" <- w95
              }
              "xalpha vertical peak diff" <- w48
              n35 = for {
                tunnel: [w90] -> w46
                tunnel: w48 -> [w77] mode=indexing
                tunnel: w49 -> [w80] mode=indexing
                tunnel: [w75] -> w60
                tunnel: [w71] -> w47 mode=indexing
                i -> [w88]
                n36 = local read "derivative bin size 1"() -> (w87:dbl)
                n37 = Index Array(array=w90, index (dim 0)=0 ("index (vol)"), index (dim 1)=w88) -> (element=w83)  [unwired: 2 in]
                n38 = Transpose 2D Array(2D array=w83) -> (transposed array=w82:void[][])
                n39 = Divide(x=w77, y=2.0) -> (x/y=w79:dbl)
                n40 = call "Derivative (2D).vi"("Axis Array"=w87, "Conductance"=w82) -> ("Transconductance"=w81:dbl[][])  [unwired: 7 in, 2 out]
                n41 = Add(x=w80, y=w79) -> (x+y=w78:dbl)
                n42 = Transpose 2D Array(2D array=w81) -> (transposed array=w64:dbl[][])
                "xalpha Top loop Intensity Graph" <- w64
                n43 = Index Array(array=w64, index (row)=w78) -> (element=w63:dbl[])  [unwired: 1 in]
                "xalpha top loop" <- w63
                n44 = Unbundle(w75) -> ("Offset"=w69, "Multiplier"=w70)
                n45 = call <vilib>:"Peak Detector.vi"("peaks/valleys"=enum32{"Peaks", "Valleys"}."Peaks", "width"="xalpha width 2", "threshold"="xalpha threshold 2", "X"=w63) -> ("Locations"=w73:dbl[])  [unwired: 3 in, 4 out]
                n46 = Multiply(x=w73, y=w70) -> (x*y=w74:dbl[])
                n47 = Add(x=w74, y=w69) -> (x+y=w72:dbl[])
                n48 = Index Array(array=w72, index #1=0 ("index"), index #2=1 ("index")) -> (element #1=w67:dbl, element #2=w68:dbl)
                n49 = Subtract(x=w68, y=w67) -> (x-y=w71:dbl)
              }
              "xalpha Vsg?" <- w47
              n50 = Bundle(w55, w47) -> (w56:cluster{dbl[], dbl[]})  [unwired: 1 in]
              n51 = Bundle(w55, w54) -> (w58:cluster{dbl[], dbl[]})  [unwired: 1 in]
              n52 = Bundle(w54, w47) -> (→"xalpha Vsd vs Vsg":cluster{dbl[], dbl[]})  [unwired: 1 in]
              n53 = Build Array(w56, w58) -> (→"xalpha Y line cut 9":cluster{dbl[], dbl[]}[])
            }
            frame Enabled {
            }
          }
        }
      }
      n54 = local read "Fast"() -> ()  [unwired: 1 out]
      n55 = local read "Slow"() -> ()  [unwired: 1 out]
    }
    frame Enabled {
    }
  }
  n56 = call <vilib>:"Add State(s) to Queue__jki_lib_state_machine.vi"("State(s) in (\"\")"="Macro: Initialize") -> ("States Out"=w2:string)  [unwired: 14 in]
  n57 = while "JKI State Machine 2018" {
    shift-right: [w122] -> _
    shift-left: _ -> [w118]
    shift-right: [w125] -> _
    shift-left: _ -> [w120]
    shift-right: [w124] -> _
    shift-left: w2 -> [w126]
    stop <- w123 stop-if-true
    w121 = -1  # Timeout
    # "Template Copyright © 2018 JKI - http://jki.net/state-machine"
    n58 = call <vilib>:"Parse State Queue__jki_lib_state_machine.vi"("State Queue"=w126, "Error In (no error)"=w120) -> ("Remaining States"=w128:string, "Current State"=w119:string, "Arguments"=w127:string)  [unwired: 11 in]
    "Status" <- w119
    n59 = case shown="\"Data Visualize: XY Graphs\"" w119 {
      selector: w119 -> [_ _ w224 _ _ _ _ _ _ _ _ _ _ _ _ _ _ _ _ _ _ w524 _ _ _ _ _ _ _ _ _ _ _ _ _ _ _ _ _ _ _ _ _ _ _ _ _ _ _ _ _ _]
      tunnel: w128 -> [w135 w223 w228 w247 w249 w257 w261 w283 w289 w307 w330 w334 w357 w372 w393 w406 w410 w419 w439 w445 w456 w527 w535 w540 w551 w555 w561 w566 w570 w585 w594 w617 w628 w632 w648 w668 w674 w688 w707 w743 w785 w814 w857 w893 w918 w953 w971 w1045 w1098 w1148 w1174 w1183]
      tunnel: w127 -> [_ _ _ _ _ _ _ _ _ _ _ _ _ _ _ _ _ _ _ w440 w451 _ _ _ _ _ _ _ _ _ _ _ _ _ _ _ _ _ _ _ _ _ _ _ _ _ _ _ _ _ _ _]
      tunnel: [w132 w221 w230 w245 errorcluster {"status"=FALSE, "code"=0, "source"=""} ("error out") w253 w259 w280 w285 w300 w309 w332 w348 w361 w373 w395 w408 w415 w437 w441 w453 w525 w533 w538 w549 w553 w559 w564 w568 w583 w590 w615 w625 w630 w646 w662 w672 w686 w705 w741 w783 w816 w850 w886 w912 w937 w969 w1038 w1091 w1144 w1172 w1180] -> w125
      tunnel: w120 -> [w131 w221 w229 w245 w250 w253 w259 w280 w286 w304 w310 w332 _ w362 w377 w396 w408 w412 w437 w442 w454 w525 w533 w538 w549 w553 w559 w564 w568 w583 w589 w615 w626 w630 w633 w662 w672 w686 w696 w737 w777 w808 w850 w885 w912 w943 w969 w1026 w1079 w1144 w1172 w1178]
      tunnel: [w134 w222 w227 w246 w252 w256 w260 w282 w288 w306 w329 w333 w356 w371 w392 w405 w409 w418 w438 w444 w455 w526 w534 w539 w550 w554 w560 w565 w569 w584 w593 w616 w627 w631 w647 w667 w673 w687 w706 w742 w784 w819 w859 w892 w917 w952 w970 w1044 w1097 w1147 w1173 w1182] -> w124
      tunnel: [_ _ _ _ _ TRUE _ _ _ _ _ _ _ _ _ _ _ _ _ _ _ _ _ _ _ _ _ _ _ _ _ _ _ _ _ _ _ _ _ _ _ _ _ _ _ _ _ _ _ _ _ _] -> w123
      tunnel: [w130 w220 w226 w235 w248 w254 w258 w281 w284 w291 w313 w331 w339 w370 w391 w404 w407 w411 w420 w443 w450 w523 w532 w536 w541 w552 w558 w562 w567 w575 w587 w614 w618 w629 w634 w661 w671 w675 w698 w733 w772 w813 w856 w890 w910 w942 w955 w1043 w1082 w1132 w1171 w1175] -> w122
      tunnel: w121 -> [w129 _ _ _ _ _ _ _ _ _ _ _ _ _ _ _ _ _ _ _ _ _ _ _ _ _ _ _ _ _ _ _ _ _ _ _ _ _ _ _ _ _ _ _ _ _ _ _ _ _ _ _]
      tunnel: w118 -> [w133 w220 w226 w236 w248 w254 w258 _ w284 w290 w313 w331 w340 w370 w391 w404 w407 w411 w420 w443 w450 w523 w532 w536 w541 w552 w558 w562 w567 w576 w588 w614 w618 w629 w635 w656 w671 w675 w699 w732 w773 w809 w851 w891 w911 w935 w955 w1043 w1082 w1132 w1171 w1175]
      frame "", "Event Structure", "Idle" {
        # "executes when the state queue is empty"
        n60 = event shown="[7] \"Cursor Graph\": Cursor Move;  \"Tab Control\", \"XY Data\": Value Change" {
          selector: _ -> [_ _ _ _ _ _ _ _ _ _ _ _ _]
          dyn-events: _ -> [_ _ _ _ _ _ _ _ _ _ _ _ _]
          timeout: w129 -> [_ _ _ _ _ _ _ _ _ _ _ _ _]
          tunnel: w135 -> [w139 w144 w150 w156 w162 w168 w176 w184 w193 w198 w203 w211 w219]
          tunnel: [w138 w143 w149 w155 w161 w167 w175 w183 w192 w197 w202 w210 w218] -> w134
          tunnel: w133 -> [w136 w141 w147 w153 w159 w165 w173 w181 w190 w195 w200 w208 w216]
          tunnel: [w137 w142 w148 w154 w160 w166 w174 w182 w191 w196 w201 w209 w217] -> w132
          tunnel: w131 -> [w137 w142 w148 w154 w160 w166 w174 w182 w191 w196 w201 w209 w217]
          tunnel: [w136 w141 w147 w153 w159 w165 w173 w181 w190 w195 w200 w208 w216] -> w130
          event Timeout {
            n61 = event-data() -> ()  [unwired: 1 in, 1 out]
            n62 = call <vilib>:"Add State(s) to Queue__jki_lib_state_machine.vi"("State(s) in (\"\")"=w139) -> ("States Out"=w138:string)  [unwired: 14 in]
          }
          event "OK": Value Change {
            # "Exit Button Value Change (pressed) Event\n(this executes Macro: Exit to terminate the VI)"
            n63 = event-data() -> ()  [unwired: 1 in, 6 out]
            n64 = call <vilib>:"Add State(s) to Queue__jki_lib_state_machine.vi"("State(s) in Front (\"\")"="Macro: Exit", "State(s) in (\"\")"=w144) -> ("States Out"=w143:string)  [unwired: 13 in]
          }
          event Panel Close? {
            # "Discard the event because we'll close the front panel ourselves in Macro: Exit"
            # "Close Panel button (pressed) Event\n(this executes Macro: Exit to terminate the VI)"
            n65 = event-data() -> ()  [unwired: 1 in, 1 out]
            n66 = call <vilib>:"Add State(s) to Queue__jki_lib_state_machine.vi"("State(s) in Front (\"\")"="Macro: Exit", "State(s) in (\"\")"=w150) -> ("States Out"=w149:string)  [unwired: 13 in]
            n67 = event-data("Discard?"=TRUE) -> ()  [unwired: 1 in, 1 out]
          }
          event "Visualize Button": Value Change {
            # "Visualize button (pressed) Event\n(this executes Macro: Visualize to load new data and plot"
            n68 = event-data() -> ()  [unwired: 1 in, 6 out]
            n69 = local write "Visualize Button"(FALSE ("Visualize Button")) -> ()
            n70 = call <vilib>:"Add State(s) to Queue__jki_lib_state_machine.vi"("State(s) in Front (\"\")"="Macro: Visualize", "State(s) in (\"\")"=w156) -> ("States Out"=w155:string)  [unwired: 13 in]
          }
          event "Check Files Button": Value Change {
            # "Visualize button (pressed) Event\n(this executes Macro: Visualize to load new data and plot"
            n71 = event-data() -> ()  [unwired: 1 in, 6 out]
            n72 = local write "Check Files Button"(FALSE ("Visualize Button")) -> ()
            n73 = call <vilib>:"Add State(s) to Queue__jki_lib_state_machine.vi"("State(s) in Front (\"\")"="Data Generation: Check Files", "State(s) in (\"\")"=w162) -> ("States Out"=w161:string)  [unwired: 13 in]
          }
          event "Generate Button": Value Change {
            # "Visualize button (pressed) Event\n(this executes Macro: Visualize to load new data and plot"
            n74 = event-data() -> ()  [unwired: 1 in, 6 out]
            n75 = local write "Generate Button"(FALSE ("Generate Button")) -> ()
            n76 = call <vilib>:"Add State(s) to Queue__jki_lib_state_machine.vi"("State(s) in Front (\"\")"="Macro: Generate", "State(s) in (\"\")"=w168) -> ("States Out"=w167:string)  [unwired: 13 in]
          }
          event "Export ITX": Value Change {
            w172 = "UI: Cursor Set >> Busy\nData Export: Export"  # UI: Cursor Set >> Busy Data Export: Export
            # "Close Panel button (pressed) Event\n(this executes Macro: Exit to terminate the VI)"
            n77 = event-data() -> ()  [unwired: 1 in, 6 out]
            n78 = local write "Export ITX"(FALSE ("Export")) -> ()
            n79 = call <vilib>:"Add State(s) to Queue__jki_lib_state_machine.vi"("State(s) in Front (\"\")"=w172, "State(s) at Back (\"\")"="UI: Cursor Set >> Idle") -> ("States Out"=w171:string)  [unwired: 13 in]
            n80 = call <vilib>:"Add State(s) to Queue__jki_lib_state_machine.vi"("State(s) in Front (\"\")"=w171, "State(s) in (\"\")"=w176) -> ("States Out"=w175:string)  [unwired: 13 in]
          }
          event "Cursor Graph": Cursor Move; "Tab Control": Value Change {
            # "Close Panel button (pressed) Event\n(this executes Macro: Exit to terminate the VI)"
            n81 = event-data() -> ()  [unwired: 1 in, 4 out]
            n82 = local read "Tab Control"() -> (w180:T1)
            n83 = case shown="\"XY Graphs\"" w180 {
              tunnel: ["" "Data Visualize: XY Graphs" "Data Visualize: Choose Data 1\nData Visualize: Choose Data 2\nGraph: Linecuts" "Data Visualize: 3D"] -> w178
              frame Default {
              }
              frame "XY Graphs" {
              }
              frame "Intensity Graphs" {
              }
              frame "3D" {
              }
            }
            n84 = call <vilib>:"Add State(s) to Queue__jki_lib_state_machine.vi"("State(s) in Front (\"\")"="Data Visualize: Calculate Indices", "State(s) in (\"\")"=w178) -> ("States Out"=w179:string)  [unwired: 13 in]
            n85 = call <vilib>:"Add State(s) to Queue__jki_lib_state_machine.vi"("State(s) in Front (\"\")"=w179, "State(s) in (\"\")"=w184) -> ("States Out"=w183:string)  [unwired: 13 in]
          }
          event "x3D Graph 9", "x3D Graph 10": Cursor Move; Value Change {
            # "Close Panel button (pressed) Event\n(this executes Macro: Exit to terminate the VI)"
            n86 = event-data() -> ()  [unwired: 1 in, 4 out]
            n87 = call <vilib>:"Add State(s) to Queue__jki_lib_state_machine.vi"("State(s) in Front (\"\")"="Data Visualize: 3D", "State(s) in (\"\")"=w193) -> ("States Out"=w192:string)  [unwired: 13 in]
          }
          event "Intensity Graph 1": Cursor Move {
            # "Close Panel button (pressed) Event\n(this executes Macro: Exit to terminate the VI)"
            n88 = event-data() -> ()  [unwired: 1 in, 9 out]
            n89 = call <vilib>:"Add State(s) to Queue__jki_lib_state_machine.vi"("State(s) in Front (\"\")"="Graph: Linecuts", "State(s) in (\"\")"=w198) -> ("States Out"=w197:string)  [unwired: 13 in]
          }
          event "Intensity Graph 2": Cursor Move {
            # "Close Panel button (pressed) Event\n(this executes Macro: Exit to terminate the VI)"
            n90 = event-data() -> ()  [unwired: 1 in, 9 out]
            n91 = call <vilib>:"Add State(s) to Queue__jki_lib_state_machine.vi"("State(s) in Front (\"\")"="Graph: Linecuts", "State(s) in (\"\")"=w203) -> ("States Out"=w202:string)  [unwired: 13 in]
          }
          event "fake point 1", "e^2/h? 1", "Log scale? 1", "derivative bin size 1", "X Offset 1": Value Change {
            # "Close Panel button (pressed) Event\n(this executes Macro: Exit to terminate the VI)"
            n92 = event-data() -> ()  [unwired: 1 in, 6 out]
            n93 = call <vilib>:"Add State(s) to Queue__jki_lib_state_machine.vi"("State(s) in Front (\"\")"="UI: Cursor Set >> Busy\nGraph: Set Labels\nData Visualize: Calculate Indices", "State(s) in (\"\")"="Data Visualize: Choose Data 1\n//Data Visualize: Choose Data 2\nGraph: Linecuts", "State(s) at Back (\"\")"="UI: Cursor Set >> Idle") -> ("States Out"=w206:string)  [unwired: 12 in]
            n94 = call <vilib>:"Add State(s) to Queue__jki_lib_state_machine.vi"("State(s) in Front (\"\")"=w206, "State(s) in (\"\")"=w211) -> ("States Out"=w210:string)  [unwired: 13 in]
          }
          event "fake point 2", "e^2/h? 2", "Log scale? 2", "derivative bin size 2", "X Offset 2": Value Change {
            # "Close Panel button (pressed) Event\n(this executes Macro: Exit to terminate the VI)"
            n95 = event-data() -> ()  [unwired: 1 in, 6 out]
            n96 = call <vilib>:"Add State(s) to Queue__jki_lib_state_machine.vi"("State(s) in Front (\"\")"="UI: Cursor Set >> Busy\nGraph: Set Labels\nData Visualize: Calculate Indices", "State(s) in (\"\")"="//Data Visualize: Choose Data 1\nData Visualize: Choose Data 2\nGraph: Linecuts", "State(s) at Back (\"\")"="UI: Cursor Set >> Idle") -> ("States Out"=w215:string)  [unwired: 12 in]
            n97 = call <vilib>:"Add State(s) to Queue__jki_lib_state_machine.vi"("State(s) in Front (\"\")"=w215, "State(s) in (\"\")"=w219) -> ("States Out"=w218:string)  [unwired: 13 in]
          }
        }
      }
      frame "---------- Core ----------" {
        # "Do not put any code in this frame.\n(it is a separator no-op)"
        n98 = call <vilib>:"Add State(s) to Queue__jki_lib_state_machine.vi"("State(s) in (\"\")"=w223) -> ("States Out"=w222:string)  [unwired: 14 in]
      }
      frame Default {
        w233 = 42 items=["No error", "Argument error", "Memory is full", "Out of zone", "End of file", "File already open", "Generic file I/O error", "File not found", "File permission error", "Disk is full", "Duplicate path", "Too many files open", "System feature not enabled", "Resource file not found", "Cannot add resource", "Resource not found", "Image not found", "Image memory error", "Pen does not exist", "Config type invalid", "Config token not found", "Config parse error", "Config memory error", "Bad external code format", "Bad external code offset", "External code not present", "Null window", "Destroy window error", "Null menu", "Print aborted", "Bad print record", "Print driver error", "Windows error during printing", "Memory error during printing", "Print dialog error", "Generic print error", "Invalid device refnum", "Device not found", "Device parameter error", "Device unit error", "Cannot open device", "Device call aborted", "Generic error", "Cancelled by user", "Object ID too low", "Object ID too high", "Object not in heap", "Unknown heap", "Unknown object (invalid DefProc)", "Unknown object (DefProc not in table)", "Message out of range", "Invalid (null) method", "Unknown message", "Manager call not supported", "Bad address", "Network operation in progress", "Network operation timed out", "Connection is busy", "Network attribute not supported", "Network error", "Address in use", "System out of memory", "Connection aborted", "Connection refused", "Not connected", "Already connected", "Connection closed", "Initialization error (interapplication manager)", "Bad occurrence", "Wait on unbound occurrence handler", "Occurrence queue overflow", "Datalog type conflict", "Unused", "Unrecognized type (interapplication manager)", "Memory corrupt", "Failed to make temporary DLL", "Old CIN version", "Drag socket not found", "Failed to load drop-object", "Failed to register OLE object", "Failed to release OLE object", "Format specifier type mismatch", "Unknown format specifier", "Too few format specifiers", "Too many format specifiers", "Scan failed", "Newer CIN version", "Error converting to variant", "Runtime menu error", "Password tampered", "Variant attribute not found", "Incompatible variant data type", "Event data is not available", "Event Store is not present", "Occurrence is not found", "Event Queue is not created", "Event info is not available", "Refnum passed is NULL", "Error retrieving Class GUID", "Error retrieving CoClass GUID", "Error retrieving TypeLib GUID.", "Bad built application magic bytes.", "Specific driver is different from the specific driver associated with the Logical Name.", "There is no session opened to the class driver.", "Max Error", "MAX - Error with config objects", "MAX - Error loading configuration", "MAX - Group not supported"]
        # "Current State"
        # "Do not delete, rename, or modify this frame.\n(this is used to capture unhandled states and typos)"
        # "Handle mistyped state name (developer tool)"
        n99 = Format Into String(format string="Software Exception: Unhandled State \"%s\"." ("message"), error in=w229, w224) -> (resulting string=w232:string, error out=w231:errorcluster)  [unwired: 1 in]
        n100 = call <vilib>:"Error Cluster From Error Code.vi"("show call chain? (False)"=TRUE, "error in (no error)"=w231, "error message (\"\")"=w232, "error code (0)"=w233) -> ("error out"=w230:errorcluster)  [unwired: 5 in]
        n101 = call <vilib>:"Add State(s) to Queue__jki_lib_state_machine.vi"("State(s) in (\"\")"=w228) -> ("States Out"=w227:string)  [unwired: 14 in]
      }
      frame "Initialize Core Data" {
        # "Do not delete, rename, or modify this frame.\n(this is used to determine panel behavior on exit)"
        # "originally closed?"
        # "exe?"
        # "If panel starts closed or is an EXE, then close it when we exit"
        n102 = property class="VI"() -> ("FP.State"=w239:T12)  [unwired: 2 in, 2 out]
        n103 = property class="App"() -> ("App.Kind"=w244:T13)  [unwired: 2 in, 2 out]
        n104 = control-ref of="Current VI Reference"() -> (w240:refnum<vi>)
        n105 = Equal?(x=w239, y=T12."Closed" ("Front Panel Window:State")) -> (x = y?=w237:bool)
        n106 = Equal?(x=w244, y=T13."Run Time System" ("Application:Kind")) -> (x = y?=w242:bool)
        n107 = Or(x=w237, y=w242) -> (x .or. y?=w241:bool)
        n108 = Bundle By Name(cluster=w236, "Core.Current VI Reference"=w240, "Core.Close Panel on Exit?"=w241) -> (w235:T15)
        n109 = call <vilib>:"Add State(s) to Queue__jki_lib_state_machine.vi"("State(s) in (\"\")"=w247) -> ("States Out"=w246:string)  [unwired: 14 in]
      }
      frame "Error Handler" {
        (unwired) "/* Post Error States"
        # "continue after error"
        # "Unhandled Error -- Display it"
        # "Handle any errors here.\nYou can also output any states to clean-up after errors occur"
        # "Clear error"
        n110 = call <vilib>:"General Error Handler.vi"("error in (no error)"=w250) -> ()  [unwired: 10 in, 5 out]
        n111 = call <vilib>:"Add State(s) to Queue__jki_lib_state_machine.vi"("State(s) in (\"\")"=w249) -> ("States Out"=w252:string)  [unwired: 14 in]
      }
      frame "Exit" {
        # "Do not put any code in this frame.\n(No errors that occur here will be handled.)"
        n112 = call <vilib>:"Add State(s) to Queue__jki_lib_state_machine.vi"("State(s) in (\"\")"=w257) -> ("States Out"=w256:string)  [unwired: 14 in]
      }
      frame "---------- Data ----------" {
        # "Do not put any code in this frame.\n(It is a separator no-op. You can make a copy of this frame to create a new Data frame)"
        n113 = call <vilib>:"Add State(s) to Queue__jki_lib_state_machine.vi"("State(s) in (\"\")"=w261) -> ("States Out"=w260:string)  [unwired: 14 in]
      }
      frame "Data: Initialize" {
        w264 = dbl[] []  # V2T
        w272 = T14 {"Open DAT Path"=path "", "Export ITX Path"=path "", "Export ITX Name"="", "Intensity 1"=enum."IV-4T", "X Offset 1"=0.0, "derivative bin size 1"=0.0, "e^2/h? 1"=FALSE, "Log scale? 1"=FALSE, "fake point 1"=0.0, "Intensity 2"=enum."IV-4T", "X Offset 2"=0.0, "derivative bin size 2"=0.0, "e^2/h? 2"=FALSE, "Log scale? 2"=FALSE, "fake point 2"=0.0}  # INI
        w275 = refnum<class "Configuration.lvclass"> refnum  # Configuration
        w276 = T16 {"Intensity 1"=refnum, "V 1"=refnum, "H 1"=refnum, "Intensity 2"=refnum, "V 2"=refnum, "H 2"=refnum}  # Graph
        w262 = 0  # Column
        w268 = dbl[] []  # Vslow Slice
        w269 = dbl[] []  # Vfast Slice
        w263 = 0  # Row
        w265 = i32[] []  # Column []
        w266 = i32[] []  # Row []
        w267 = 0  # Page
        w277 = T17 {"IV-4T"=[], "IV-2T"=[], "G-4T"=[], "R-4T"=[], "G-2T"=[], "R-2T"=[], "dG-4T"=[], "Differential Mode"=[], "Common Mode"=[]}  # 3D
        w270 = string[] []  # Scan Names
        w271 = dbl[] []  # Vslowest
        w273 = dbl[] []  # Vslow
        w278 = dbl[][] []  # Vfast
        w274 = refnum<class "Retrieve and Visualize.lvclass"> refnum  # R&V
        w279 = T18 {"Current VI Reference"=refnum, "Close Panel on Exit?"=FALSE}  # Core
        # "Initialize the shift-register data, here.\n(data names are defined by what you wire into the bundle function)"
        n114 = Bundle("Core"=w279, "R&V"=w274, "Configuration"=w275, "INI"=w272, "3D"=w277, "Graph"=w276, "Vfast"=w278, "Vslow"=w273, "Vslowest"=w271, "Scan Names"=w270, "Vfast Slice"=w269, "Vslow Slice"=w268, "Page"=w267, "Row"=w263, "Column"=w262, "Row []"=w266, "Column []"=w265, "V2T"=w264) -> (w281:T15)  [unwired: 1 in]
        n115 = call <vilib>:"Add State(s) to Queue__jki_lib_state_machine.vi"("State(s) in (\"\")"=w283) -> ("States Out"=w282:string)  [unwired: 14 in]
      }
      frame "Data: Cleanup" {
        # "Cleanup any data and references, here.\n(this is called automatically, by the Macro: Exit)"
        n116 = Unbundle By Name(w284) -> ("Core.Current VI Reference"=w287:refnum<vi>)
        n117 = Close Reference(reference=w287, error in (no error)=w286) -> (error out=w285:errorcluster)
        n118 = call <vilib>:"Add State(s) to Queue__jki_lib_state_machine.vi"("State(s) in (\"\")"=w289) -> ("States Out"=w288:string)  [unwired: 14 in]
      }
      frame "Data: Read INI" {
        w298 = T19 3 items=["User Home"=0, "User Desktop"=1, "User Documents"=2, "User Application Data"=3, "User Preferences"=4, "User Temporary"=5, "Public Documents"=6, "Public Application Data"=7, "Public Preferences"=8, "Public Cache"=13, "System Core Libraries"=9, "System Installed Libraries"=10, "Application Files"=11, "Boot Volume Root"=12] ("system directory type")
        # "Do not put any code in this frame.\n(It is a separator no-op. You can make a copy of this frame to create a new Data frame)"
        n119 = Unbundle By Name(w290) -> ("Configuration"=w292:refnum<class "Configuration.lvclass">, "INI"=w293:T14)
        n120 = call <vilib>:"Get System Directory.vi"("system directory type"=w298) -> ("system directory"=w295:path)  [unwired: 10 in]
        n121 = Build Path(base path=w295, name or relative path="LevyLab\\Retrieve and Visualize") -> (appended path=w297:path)
        n122 = call <userlib>:"Write Path.vi"("error in (no error)"=w304, "Path"=w297, "Configuration in"=w292) -> ("error out"=w303:errorcluster, "Configuration out"=w305:refnum<class "Configuration.lvclass">)  [unwired: 7 in]
        n123 = call <userlib>:"Read Configuration.vi"("INI Fomatted Cluster Type"=w293, "error in (no error)"=w303, "Configuration in"=w305) -> ("error out"=w301:errorcluster, "Configuration"=w302:variant, "Configuration out"=w299:refnum<class "Configuration.lvclass">)  [unwired: 6 in]
        n124 = Variant To Data(error in=w301, type=w293, Variant=w302) -> (data=w296:T14, error out=w300:errorcluster)
        n125 = Bundle By Name(cluster=w290, "Configuration"=w299, "INI"=w296) -> (w291:T15)
        n126 = call <vilib>:"Add State(s) to Queue__jki_lib_state_machine.vi"("State(s) in (\"\")"=w307) -> ("States Out"=w306:string)  [unwired: 14 in]
      }
      frame "Data: Write INI" {
        # "Do not put any code in this frame.\n(It is a separator no-op. You can make a copy of this frame to create a new Data frame)"
        n127 = local read "fake point 2"() -> (w314:dbl)
        n128 = local read "Open DAT Path"() -> (w328:path)
        n129 = local read "Export ITX Path"() -> (w327:path)
        n130 = local read "Export ITX Name"() -> (w326:string)
        n131 = local read "Intensity 1"() -> (w325:T7)
        n132 = local read "X Offset 1"() -> (w324:dbl)
        n133 = local read "derivative bin size 1"() -> (w323:dbl)
        n134 = local read "e^2/h? 1"() -> (w322:bool)
        n135 = local read "Log scale? 1"() -> (w321:bool)
        n136 = local read "fake point 1"() -> (w320:dbl)
        n137 = local read "Intensity 2"() -> (w319:T7)
        n138 = local read "X Offset 2"() -> (w318:dbl)
        n139 = local read "derivative bin size 2"() -> (w317:dbl)
        n140 = local read "e^2/h? 2"() -> (w316:bool)
        n141 = local read "Log scale? 2"() -> (w315:bool)
        n142 = Unbundle By Name(w313) -> ("Configuration"=w312:refnum<class "Configuration.lvclass">, "INI"=w308:T14)
        n143 = Bundle By Name(cluster=w308, "Open DAT Path"=w328, "Export ITX Path"=w327, "Export ITX Name"=w326, "Intensity 1"=w325, "X Offset 1"=w324, "derivative bin size 1"=w323, "e^2/h? 1"=w322, "Log scale? 1"=w321, "fake point 1"=w320, "Intensity 2"=w319, "X Offset 2"=w318, "derivative bin size 2"=w317, "e^2/h? 2"=w316, "Log scale? 2"=w315, "fake point 2"=w314) -> (w311:T14)
        n144 = call <userlib>:"Write Configuration.vi"("error in (no error)"=w310, "Variant"=w311, "Configuration in"=w312) -> ("error out"=w309:errorcluster)  [unwired: 7 in, 1 out]
        n145 = call <vilib>:"Add State(s) to Queue__jki_lib_state_machine.vi"("State(s) in (\"\")"=w330) -> ("States Out"=w329:string)  [unwired: 14 in]
      }
      frame "---------- Graph ----------" {
        # "Do not put any code in this frame.\n(It is a separator no-op. You can make a copy of this frame to create a new Data frame)"
        n146 = call <vilib>:"Add State(s) to Queue__jki_lib_state_machine.vi"("State(s) in (\"\")"=w334) -> ("States Out"=w333:string)  [unwired: 14 in]
      }
      frame "Graph: Initialize" {
        # "Do not put any code in this frame.\n(It is a separator no-op. You can make a copy of this frame to create a new Data frame)"
        n147 = control-ref of="Intensity Graph 1"() -> (w355:refnum<vi>)
        n148 = control-ref of="H Cut 1"() -> (w338:refnum<vi>)
        n149 = control-ref of="V Cut 1"() -> (w337:refnum<vi>)
        n150 = control-ref of="Intensity Graph 2"() -> (w341:refnum<vi>)
        n151 = control-ref of="H Cut 2"() -> (w336:refnum<vi>)
        n152 = control-ref of="V Cut 2"() -> (w335:refnum<vi>)
        n153 = call <userlib>:"Write Intensity Graph ref.vi"("Intensity Graph (Control)"=w355, "Intensity Graph"=w355) -> ("error out"=w345:errorcluster, "graph_utilities out"=w354:refnum<class "graph_utilities.lvclass">)  [unwired: 8 in]
        n154 = call <userlib>:"Write Intensity Graph ref.vi"("Intensity Graph (Control)"=w341, "Intensity Graph"=w341) -> ("error out"=w344:errorcluster, "graph_utilities out"=w351:refnum<class "graph_utilities.lvclass">)  [unwired: 8 in]
        n155 = call <userlib>:"Write XY Graph ref.vi"("XY Graph (Control)"=w338, "XY Graph"=w338, "graph_utilities in"=w354) -> ("error out"=w346:errorcluster, "graph_utilities out"=w353:refnum<class "graph_utilities.lvclass">)  [unwired: 7 in]
        n156 = call <userlib>:"Write XY Graph ref.vi"("XY Graph (Control)"=w336, "XY Graph"=w336, "graph_utilities in"=w351) -> ("error out"=w343:errorcluster, "graph_utilities out"=w350:refnum<class "graph_utilities.lvclass">)  [unwired: 7 in]
        n157 = call <userlib>:"Write XY Graph ref.vi"("XY Graph (Control)"=w337, "XY Graph"=w337, "graph_utilities in"=w354) -> ("error out"=w347:errorcluster, "graph_utilities out"=w352:refnum<class "graph_utilities.lvclass">)  [unwired: 7 in]
        n158 = call <userlib>:"Write XY Graph ref.vi"("XY Graph (Control)"=w335, "XY Graph"=w335, "graph_utilities in"=w351) -> ("error out"=w342:errorcluster, "graph_utilities out"=w349:refnum<class "graph_utilities.lvclass">)  [unwired: 7 in]
        n159 = Bundle By Name(cluster=w340, "Graph.Intensity 1"=w354, "Graph.H 1"=w353, "Graph.V 1"=w352, "Graph.Intensity 2"=w351, "Graph.H 2"=w350, "Graph.V 2"=w349) -> (w339:T15)
        n160 = Merge Errors(w345, w346, w347, w344, w343, w342) -> (w348:errorcluster)
        n161 = call <vilib>:"Add State(s) to Queue__jki_lib_state_machine.vi"("State(s) in (\"\")"=w357) -> ("States Out"=w356:string)  [unwired: 14 in]
      }
      frame "Graph: Set Y" {
        # "Do not put any code in this frame.\n(It is a separator no-op. You can make a copy of this frame to create a new Data frame)"
        n162 = Unbundle By Name(w370) -> ("Graph.Intensity 1"=w369:refnum<class "graph_utilities.lvclass">, "Graph.Intensity 2"=w368:refnum<class "graph_utilities.lvclass">, "Scan Names"=w360:string[], "Vfast Slice"=w358:dbl[])  [unwired: 1 out]
        n163 = Index Array(array=w360) -> (element=w359:string)  [unwired: 1 in]
        n164 = call <userlib>:"Set Intensity Graph Y Label.vi"("error in (no error)"=w362, "Y Label"=w359, "graph_utilities in"=w369) -> ("error out"=w366:errorcluster, "graph_utilities out"=w365:refnum<class "graph_utilities.lvclass">)  [unwired: 7 in]
        n165 = call <userlib>:"Set Intensity Graph Y Scale Array.vi"("error in (no error)"=w366, "Y Scale"=w358, "graph_utilities in"=w365) -> ("error out"=w364:errorcluster)  [unwired: 7 in, 1 out]
        n166 = call <userlib>:"Set Intensity Graph Y Label.vi"("error in (no error)"=w364, "Y Label"=w359, "graph_utilities in"=w368) -> ("error out"=w363:errorcluster, "graph_utilities out"=w367:refnum<class "graph_utilities.lvclass">)  [unwired: 7 in]
        n167 = call <userlib>:"Set Intensity Graph Y Scale Array.vi"("error in (no error)"=w363, "Y Scale"=w358, "graph_utilities in"=w367) -> ("error out"=w361:errorcluster)  [unwired: 7 in, 1 out]
        n168 = call <vilib>:"Add State(s) to Queue__jki_lib_state_machine.vi"("State(s) in (\"\")"=w372) -> ("States Out"=w371:string)  [unwired: 14 in]
      }
      frame "Graph: Set Labels" {
        w379 = string[][] [["IV", "I (A)", "V_4T (V)"], ["IV-2T", "I (A)", "V_2T (V)"], ["d/dx(IV) R", "I (A)", "R (ohms)"], ["d/dy(IV) G", "V_4T (V)", "G (S)"], ["d/dx(IV-2T) R", "I (A)", "R (ohms)"], ["d/dy(IV-2T) G", "V_2T (V)", "G (S)"], ["d2/dy2(IV) dG/dVsg", "V_4T (V)", "dG/dVbg"], ["d2/dx2(IV) dR/dI", "V_2T (V)", "dG/dVbg"]]
        # "Z scale"
        # "x scale"
        # "data"
        # "Z Scale & Label"
        # "X Scale & Label"
        # "Data Choice"
        # "Do not put any code in this frame.\n(It is a separator no-op. You can make a copy of this frame to create a new Data frame)"
        n169 = Unbundle By Name(w391) -> ("Graph.Intensity 1"=w390:refnum<class "graph_utilities.lvclass">, "Graph.Intensity 2"=w387:refnum<class "graph_utilities.lvclass">)
        n170 = Index Array(array=w379, index (row)="Intensity 2") -> (element=w385:string[])  [unwired: 1 in]
        n171 = Index Array(array=w379, index (row)="Intensity 1") -> (element=w386:string[])  [unwired: 1 in]
        n172 = Index Array(array=w386) -> (element #2=w382:string, element #3=w381:string)  [unwired: 3 in, 1 out]
        n173 = Index Array(array=w385) -> (element #2=w380:string, element #3=w378:string)  [unwired: 3 in, 1 out]
        n174 = call <userlib>:"Set Intensity Graph X Label.vi"("error in (no error)"=w377, "X Label"=w382, "graph_utilities in"=w390) -> ("error out"=w376:errorcluster, "graph_utilities out"=w389:refnum<class "graph_utilities.lvclass">)  [unwired: 7 in]
        n175 = call <userlib>:"Set Intensity Graph Z Label.vi"("error in (no error)"=w376, "Z Label"=w381, "graph_utilities in"=w389) -> ("error out"=w375:errorcluster)  [unwired: 7 in, 1 out]
        n176 = call <userlib>:"Set Intensity Graph X Label.vi"("error in (no error)"=w375, "X Label"=w380, "graph_utilities in"=w387) -> ("error out"=w374:errorcluster, "graph_utilities out"=w388:refnum<class "graph_utilities.lvclass">)  [unwired: 7 in]
        n177 = call <userlib>:"Set Intensity Graph Z Label.vi"("error in (no error)"=w374, "Z Label"=w378, "graph_utilities in"=w388) -> ("error out"=w373:errorcluster)  [unwired: 7 in, 1 out]
        n178 = call <vilib>:"Add State(s) to Queue__jki_lib_state_machine.vi"("State(s) in (\"\")"=w393) -> ("States Out"=w392:string)  [unwired: 14 in]
      }
      frame "Graph: Linecuts" {
        # "Do not put any code in this frame.\n(It is a separator no-op. You can make a copy of this frame to create a new Data frame)"
        n179 = Unbundle By Name(w404) -> ("Graph.V 1"=w403:refnum<class "graph_utilities.lvclass">, "Graph.H 1"=w400:refnum<class "graph_utilities.lvclass">, "Graph.V 2"=w401:refnum<class "graph_utilities.lvclass">, "Graph.H 2"=w402:refnum<class "graph_utilities.lvclass">)  [unwired: 2 out]
        n180 = call <userlib>:"Intensity Graph Linecut (Vertical).vi"("error in (no error)"=w396, "graph_utilities in"=w403) -> ("error out"=w394:errorcluster)  [unwired: 8 in, 1 out]
        n181 = call <userlib>:"Intensity Graph Linecut (Horizontal).vi"("error in (no error)"=w396, "graph_utilities in"=w400) -> ("error out"=w399:errorcluster)  [unwired: 8 in, 1 out]
        n182 = call <userlib>:"Intensity Graph Linecut (Vertical).vi"("error in (no error)"=w396, "graph_utilities in"=w401) -> ("error out"=w398:errorcluster)  [unwired: 8 in, 1 out]
        n183 = call <userlib>:"Intensity Graph Linecut (Horizontal).vi"("error in (no error)"=w396, "graph_utilities in"=w402) -> ("error out"=w397:errorcluster)  [unwired: 8 in, 1 out]
        n184 = Merge Errors(w394, w399, w398, w397) -> (w395:errorcluster)
        n185 = call <vilib>:"Add State(s) to Queue__jki_lib_state_machine.vi"("State(s) in (\"\")"=w406) -> ("States Out"=w405:string)  [unwired: 14 in]
      }
      frame "---------- UI ----------" {
        # "Do not put any code in this frame.\n(It is a separator no-op. You can make a copy of this frame to create a new UI frame)"
        n186 = call <vilib>:"Add State(s) to Queue__jki_lib_state_machine.vi"("State(s) in (\"\")"=w410) -> ("States Out"=w409:string)  [unwired: 14 in]
      }
      frame "UI: Initialize" {
        # "Initialize the User Interface, here.\n(this is called automatically, by the Macro: Init)"
        n187 = Unbundle By Name(w411) -> ("Core.Current VI Reference"=w413:refnum<vi>)
        n188 = property class="VI" props=["FP.Behavior"](reference=w413) -> ()  [unwired: 1 in, 3 out]
        n189 = local write "Field/Temperature"(0 ("Field/Temperature")) -> ()
        n190 = local write "OK"(FALSE ("OK")) -> ()
        n191 = call <userlib>:"Fit VI window to Largest Dec__ogtk.vi"("error in (no error)"=w412, "border spacing (2 px)"=-2) -> ("error out"=w415:errorcluster)  [unwired: 4 in, 1 out]
        n192 = call <vilib>:"Add State(s) to Queue__jki_lib_state_machine.vi"("State(s) in (\"\")"=w419) -> ("States Out"=w418:string)  [unwired: 14 in]
      }
      frame "UI: Initialize Controls" {
        # "Do not put any code in this frame.\n(It is a separator no-op. You can make a copy of this frame to create a new UI frame)"
        n193 = Unbundle By Name(w420) -> ("INI"=w421:T14)
        n194 = Unbundle By Name(w421) -> ("Open DAT Path"=w436:path, "Export ITX Path"=w435:path, "Export ITX Name"=w434:string, "Intensity 1"=w433:T7, "X Offset 1"=w432:dbl, "derivative bin size 1"=w431:dbl, "e^2/h? 1"=w430:bool, "Log scale? 1"=w429:bool, "fake point 1"=w428:dbl, "Intensity 2"=w427:T7, "X Offset 2"=w426:dbl, "derivative bin size 2"=w425:dbl, "e^2/h? 2"=w424:bool, "Log scale? 2"=w423:bool, "fake point 2"=w422:dbl)
        n195 = local write "Open DAT Path"(w436) -> ()
        n196 = local write "Export ITX Path"(w435) -> ()
        n197 = local write "Export ITX Name"(w434) -> ()
        n198 = local write "Intensity 1"(w433) -> ()
        n199 = local write "X Offset 1"(w432) -> ()
        n200 = local write "e^2/h? 1"(w430) -> ()
        n201 = local write "Log scale? 1"(w429) -> ()
        n202 = local write "fake point 1"(w428) -> ()
        n203 = local write "Intensity 2"(w427) -> ()
        n204 = local write "X Offset 2"(w426) -> ()
        n205 = local write "e^2/h? 2"(w424) -> ()
        n206 = local write "Log scale? 2"(w423) -> ()
        n207 = local write "fake point 2"(w422) -> ()
        n208 = local write "derivative bin size 1"(w431) -> ()
        n209 = local write "derivative bin size 2"(w425) -> ()
        n210 = call <vilib>:"Add State(s) to Queue__jki_lib_state_machine.vi"("State(s) in (\"\")"=w439) -> ("States Out"=w438:string)  [unwired: 14 in]
      }
      frame "UI: Cursor Set" {
        # "Argument"
        # "Set and Unset Cursor Busy.\n(Usage: \"UI: Cursor Set >> Busy|Idle\")"
        n211 = case shown="\"Idle\", Default" w440 {
          tunnel: w442 -> [w447 w449]
          tunnel: [w446 w448] -> w441
          frame "Idle", Default {
            n212 = call <vilib>:"Unset Busy.vi"("error in (no error)"=w447) -> ("error out"=w446:errorcluster)  [unwired: 10 in]
          }
          frame "Busy" {
            n213 = call <vilib>:"Set Busy.vi"("error in (no error)"=w449) -> ("error out"=w448:errorcluster)  [unwired: 9 in, 1 out]
          }
        }
        n214 = call <vilib>:"Add State(s) to Queue__jki_lib_state_machine.vi"("State(s) in (\"\")"=w445) -> ("States Out"=w444:string)  [unwired: 14 in]
      }
      frame "UI: Front Panel State" {
        # "Argument"
        # "Set Front Panel Open or Closed\n(Usage: \"UI: Front Panel State >> Open|Close\")"
        n215 = Unbundle By Name(w450) -> ("Core.Current VI Reference"=w452:refnum<vi>)
        n216 = case shown="\"Open\", \"Standard\", Default" w451 {
          tunnel: w454 -> [w462 w477 w488 w501 w514]
          tunnel: [w464 w478 w490 w503 w516] -> w453
          tunnel: w452 -> [w463 w475 w489 w502 w515]
          frame "Open", "Standard", Default {
            w457 = T12."Standard" ("State")
            n217 = property class="VI"(reference=w463, error in=w462) -> (reference out=w460:refnum<vi>, error out=w461:errorcluster, "FP.State"=w459:T12)
            n218 = Not Equal?(x=w459, y=w457) -> (x != y?=w458:bool)
            n219 = case shown="False" w458 {
              tunnel: [w468 w470] -> w464
              tunnel: w461 -> [w467 w470]
              tunnel: w460 -> [w466 _]
              tunnel: w457 -> [w465 _]
              frame True {
                n220 = invoke class="VI" method="FP.Open"(reference=w466, error in=w467, "Activate"=TRUE, "State"=w465) -> (error out=w468:errorcluster)  [unwired: 1 in, 4 out]
              }
              frame False {
              }
            }
          }
          frame "Close", "Closed" {
            n221 = property class="VI"(reference=w475, error in=w477) -> (reference out=w474:refnum<vi>, error out=w476:errorcluster, "FP.State"=w472:T12)
            n222 = Not Equal?(x=w472, y=T12."Closed" ("Front Panel Window:State")) -> (x != y?=w471:bool)
            n223 = case shown="True" w471 {
              tunnel: [w479 w482] -> w478
              tunnel: w476 -> [w479 w481]
              tunnel: w474 -> [_ w480]
              frame False {
              }
              frame True {
                n224 = invoke class="VI" method="FP.Close"(reference=w480, error in=w481) -> (error out=w482:errorcluster)  [unwired: 1 in, 2 out]
              }
            }
          }
          frame "Hidden", "Hide" {
            w483 = T12."Hidden" ("State")
            n225 = property class="VI"(reference=w489, error in=w488) -> (reference out=w486:refnum<vi>, error out=w487:errorcluster, "FP.State"=w485:T12)
            n226 = Not Equal?(x=w485, y=w483) -> (x != y?=w484:bool)
            n227 = case shown="True" w484 {
              tunnel: [w494 w495] -> w490
              tunnel: w487 -> [w493 w495]
              tunnel: w486 -> [w492 _]
              tunnel: w483 -> [w491 _]
              frame True {
                n228 = invoke class="VI" method="FP.Open"(reference=w492, error in=w493, "State"=w491) -> (error out=w494:errorcluster)  [unwired: 2 in, 4 out]
              }
              frame False {
              }
            }
          }
          frame "Minimize", "Minimized" {
            w496 = T12."Minimized" ("State")
            n229 = property class="VI"(reference=w502, error in=w501) -> (reference out=w499:refnum<vi>, error out=w500:errorcluster, "FP.State"=w498:T12)
            n230 = Not Equal?(x=w498, y=w496) -> (x != y?=w497:bool)
            n231 = case shown="True" w497 {
              tunnel: [w507 w508] -> w503
              tunnel: w500 -> [w506 w508]
              tunnel: w499 -> [w505 _]
              tunnel: w496 -> [w504 _]
              frame True {
                n232 = invoke class="VI" method="FP.Open"(reference=w505, error in=w506, "State"=w504) -> (error out=w507:errorcluster)  [unwired: 2 in, 4 out]
              }
              frame False {
              }
            }
          }
          frame "Maximize", "Maximized" {
            w509 = T12."Maximized" ("State")
            n233 = property class="VI"(reference=w515, error in=w514) -> (reference out=w512:refnum<vi>, error out=w513:errorcluster, "FP.State"=w511:T12)
            n234 = Not Equal?(x=w511, y=w509) -> (x != y?=w510:bool)
            n235 = case shown="True" w510 {
              tunnel: [w520 w521] -> w516
              tunnel: w513 -> [w519 w521]
              tunnel: w512 -> [w518 _]
              tunnel: w509 -> [w517 _]
              frame True {
                n236 = invoke class="VI" method="FP.Open"(reference=w518, error in=w519, "State"=w517) -> (error out=w520:errorcluster)  [unwired: 2 in, 4 out]
              }
              frame False {
              }
            }
          }
        }
        n237 = call <vilib>:"Add State(s) to Queue__jki_lib_state_machine.vi"("State(s) in (\"\")"=w456) -> ("States Out"=w455:string)  [unwired: 14 in]
      }
      frame "UI: Choose Tab" {
        # "Do not put any code in this frame.\n(It is a separator no-op. You can make a copy of this frame to create a new UI frame)"
        n238 = case shown="\"Intensity Graphs\", Default" w524 {
          tunnel: [T1."Intensity Graphs" ("Value (Signaling)")] -> w522
          frame "Intensity Graphs", Default {
          }
        }
        n239 = disable-structure shown="Disabled" {
          frame Disabled {
            n240 = property on="Tab Control" class="TabCtl (strict)"() -> ("Pages"=w528:refnum<vi>[])  [unwired: 2 in, 2 out]
            n241 = for {
              tunnel: w528 -> [w530] mode=indexing
              tunnel: [w529] -> _ mode=indexing
              n242 = property class="Page"(reference=w530) -> ("PageLabel"=w529:string)  [unwired: 1 in, 2 out]
            }
          }
          frame Enabled {
          }
        }
        n243 = property on="Tab Control" class="TabCtl (strict)"("Val(Sgnl)"=w522) -> ()  [unwired: 2 in, 2 out]
        n244 = call <vilib>:"Add State(s) to Queue__jki_lib_state_machine.vi"("State(s) in (\"\")"=w527) -> ("States Out"=w526:string)  [unwired: 14 in]
      }
      frame "---------- Macro ----------" {
        # "Do not put any code in this frame.\n(It is a separator no-op. You can make a copy of this frame to create a new Macro frame)"
        n245 = call <vilib>:"Add State(s) to Queue__jki_lib_state_machine.vi"("State(s) in (\"\")"=w535) -> ("States Out"=w534:string)  [unwired: 14 in]
      }
      frame "Macro: Initialize" {
        # "Initialization Macro\n(This is called once, when the VI starts)"
        n246 = call <vilib>:"Add State(s) to Queue__jki_lib_state_machine.vi"("State(s) in Front (\"\")"="Data: Initialize\nInitialize Core Data\nUI: Initialize\nUI: Front Panel State >> Open\n\nData: Read INI\nUI: Initialize Controls\n\nGraph: Initialize\nData Visualize: Initialize Graphs", "State(s) in (\"\")"=w540) -> ("States Out"=w539:string)  [unwired: 13 in]
      }
      frame "Macro: Exit" {
        # "Exit Macro\n(This is called once, when the VI exits)"
        n247 = Unbundle By Name(w541) -> ("Core.Close Panel on Exit?"=w548:bool)
        n248 = Select(t="UI: Front Panel State >> Close", s=w548, f="") -> (s? t:f=w545:string)
        n249 = call <vilib>:"Add State(s) to Queue__jki_lib_state_machine.vi"("State(s) in Front (\"\")"="Data: Write INI", "State(s) in (\"\")"=w545, "State(s) at Back (\"\")"="Data: Cleanup\nExit") -> ("States Out"=w543:string)  [unwired: 12 in]
        n250 = call <vilib>:"Add State(s) to Queue__jki_lib_state_machine.vi"("State(s) in Front (\"\")"=w543, "State(s) in (\"\")"=w551) -> ("States Out"=w550:string)  [unwired: 13 in]
      }
      frame "Macro: Update Graphs" {
        # "Do not put any code in this frame.\n(It is a separator no-op. You can make a copy of this frame to create a new Macro frame)"
        n251 = call <vilib>:"Add State(s) to Queue__jki_lib_state_machine.vi"("State(s) in (\"\")"=w555) -> ("States Out"=w554:string)  [unwired: 14 in]
      }
      frame "Macro: Visualize" {
        # "Do not put any code in this frame.\n(It is a separator no-op. You can make a copy of this frame to create a new Macro frame)"
        n252 = local write "Tab Control"(T1."Data generation" ("Tab Control")) -> ()
        n253 = call <vilib>:"Add State(s) to Queue__jki_lib_state_machine.vi"("State(s) in Front (\"\")"="Macro: Visualize", "State(s) in (\"\")"=w561) -> ("States Out"=w560:string)  [unwired: 13 in]
      }
      frame "Macro: Generate" {
        # "Do not put any code in this frame.\n(It is a separator no-op. You can make a copy of this frame to create a new Macro frame)"
        n254 = call <vilib>:"Add State(s) to Queue__jki_lib_state_machine.vi"("State(s) in Front (\"\")"="Data Generation: Update Class Wire\nData Generation: Read ITX Files\nData Generation: Write DAT File" ("State(s) in Front (\"\")"), "State(s) in (\"\")"=w566) -> ("States Out"=w565:string)  [unwired: 13 in]
      }
      frame "---------- Data Generation ----------" {
        # "Template Separator\n(You can make a copy of, or modify, this frame)"
        n255 = call <vilib>:"Add State(s) to Queue__jki_lib_state_machine.vi"("State(s) in (\"\")"=w570) -> ("States Out"=w569:string)  [unwired: 14 in]
      }
      frame "Data Generation: Update Class Wire" {
        # "Template Separator\n(You can make a copy of, or modify, this frame)"
        n256 = Unbundle By Name(w576) -> ("R&V"=w580:refnum<class "Retrieve and Visualize.lvclass">)
        n257 = Bundle By Name(cluster=w580, "File or Folder Path"="Path", "T/B third axis"="T/B third axis", "IV setup"="IV setup", "index"="index", "Portion of data"="Portion of data (%)", "Decimate point"="Decimate point", "Parameters from comments?"="Extract paramaters from comments?", "Scan names"="Scan names") -> (w574:refnum<class "Retrieve and Visualize.lvclass">)
        n258 = Bundle By Name(cluster=w576, "R&V"=w574) -> (w575:T15)
        n259 = call <vilib>:"Add State(s) to Queue__jki_lib_state_machine.vi"("State(s) in (\"\")"=w585) -> ("States Out"=w584:string)  [unwired: 14 in]
      }
      frame "Data Generation: Read ITX Files" {
        # "Your code here.\n(You can make a copy of, or modify, this frame)"
        n260 = Unbundle By Name(w588) -> ("R&V"=w592:refnum<class "Retrieve and Visualize.lvclass">)
        n261 = for {
          N: "# of fields/Temperatures" -> [w600]
          shift-right: [w607] -> w586
          shift-left: w592 -> [w604]
          tunnel: [w597] -> w590
          tunnel: w589 -> [w596]
          i -> [w599]
          n262 = Multiply(x=w599, y="Field Period") -> (x*y=w603:i32)
          n263 = Bundle By Name(cluster=w604, "# of B/T"=w600, "B/T offset"=w603, "Field Period"="Field Period") -> (w601:refnum<class "Retrieve and Visualize.lvclass">)
          n264 = call "Data retrieve engine_SE.vi"("error in (no error)"=w596, "File Type"="File Type", "Retrieve and Visualize"=w601) -> ("error out"=w606:errorcluster, "Retrieve and Visualize out"=w605:refnum<class "Retrieve and Visualize.lvclass">)  [unwired: 7 in]
          n265 = call "Create DAT Comments.vi"("error in"=w606, "Additional comments"="Additional comments", "Retrieve and Visualize"=w605) -> ("error out"=w597:errorcluster, "Retrieve and Visualize out"=w607:refnum<class "Retrieve and Visualize.lvclass">)  [unwired: 7 in]
        }
        n266 = Bundle By Name(cluster=w588, "R&V"=w586) -> (w587:T15)
        n267 = call <vilib>:"Add State(s) to Queue__jki_lib_state_machine.vi"("State(s) in (\"\")"=w594) -> ("States Out"=w593:string)  [unwired: 14 in]
      }
      frame "Data Generation: Check Files" {
        # "Template Separator\n(You can make a copy of, or modify, this frame)"
        n268 = local read "index"() -> (w608:T2)
        n269 = local read "Path"() -> (w613:path)
        n270 = local read "File Type"() -> (w612:T4)
        n271 = call "LV to ITX Retrieve_SE mode_aditi.vi"("File or Folder Path"=w613, "offset"=0, "length"=1, "index"=w608, "stop"=FALSE, "File Type"=w612) -> ()  [unwired: 3 in, 7 out]
        n272 = call <vilib>:"Add State(s) to Queue__jki_lib_state_machine.vi"("State(s) in (\"\")"=w617) -> ("States Out"=w616:string)  [unwired: 14 in]
      }
      frame "Data Generation: Write DAT File" {
        # "get file name"
        # "Your code here.\n(You can make a copy of, or modify, this frame)"
        n273 = local read "Path"() -> (w623:path)
        n274 = Strip Path(path=w623) -> (name=w621:string)  [unwired: 1 out]
        n275 = Unbundle By Name(w618) -> ("R&V"=w624:refnum<class "Retrieve and Visualize.lvclass">)
        n276 = Concatenate Strings(w621, ".dat" ("string")) -> (w619:string)
        n277 = call "Create DAT File.vi"("error in"=w626, "DAT file name"=w619, "Processed data folder"="DAT folder", "Retrieve and Visualize"=w624) -> ("error out"=w625:errorcluster)  [unwired: 6 in, 1 out]
        n278 = call <vilib>:"Add State(s) to Queue__jki_lib_state_machine.vi"("State(s) in (\"\")"=w628) -> ("States Out"=w627:string)  [unwired: 14 in]
      }
      frame "---------- Data Visualize ----------" {
        # "Template Separator\n(You can make a copy of, or modify, this frame)"
        n279 = call <vilib>:"Add State(s) to Queue__jki_lib_state_machine.vi"("State(s) in (\"\")"=w632) -> ("States Out"=w631:string)  [unwired: 14 in]
      }
      frame "Data Visualize: Read DAT File" {
        # "Template Separator\n(You can make a copy of, or modify, this frame)"
        n280 = Empty String/Path?(string/path="Open DAT Path") -> (empty?=w640:bool)
        n281 = call-poly <userlib>:"File Exists__ogtk.vi"("file path"="Open DAT Path") -> ("exists"=w642:bool)  [unwired: 6 in, 1 out]
        n282 = Not(x=w642) -> (.not. x?=w641:bool)
        n283 = Or(x=w640, y=w641) -> ()  [unwired: 1 out]
        n284 = call <vilib>:"Get File Extension.vi"("error in (no error)"=w633, "file"="Open DAT Path") -> ("error out"=w636:errorcluster, "lowercase file extension"=w639:string, "dup file"=w637:path)  [unwired: 5 in, 2 out]
        n285 = case shown="\"dat\"" w639 {
          tunnel: [w650 w653] -> w643
          tunnel: w637 -> [w650 _]
          tunnel: w636 -> [w649 w655]
          tunnel: [w649 w654] -> w644
          frame "dat" {
          }
          frame Default {
            w651 = "DAT" ("pattern label")
            n286 = call "File Dialog"("button label"=w651, "error in"=w655, "pattern (all files)"="*.dat", "pattern label"=w651) -> ("selected path"=w653:path, "error out"=w654:errorcluster)  [unwired: 8 in, 2 out]
          }
        }
        n287 = call "Read DAT File.vi"("error in"=w644, "file path (use dialog)"=w643) -> ("error out"=w646:errorcluster, "Retrieve and Visualize out"=w645:refnum<class "Retrieve and Visualize.lvclass">)  [unwired: 8 in]
        n288 = local write "Open DAT Path"(w643) -> ()
        n289 = Bundle By Name(cluster=w635, "R&V"=w645) -> (w634:T15)
        n290 = call <vilib>:"Add State(s) to Queue__jki_lib_state_machine.vi"("State(s) in (\"\")"=w648) -> ("States Out"=w647:string)  [unwired: 14 in]
      }
      frame "Data Visualize: Initialize Graphs" {
        # "IV-2T=I VS V2T"
        # "IV-4T=V4T VS V2T"
        # "take data from R&V class wire and put on\nlocal data cluster"
        # "Template Separator\n(You can make a copy of, or modify, this frame)"
        n291 = Unbundle By Name(w656) -> ("R&V"=w659:refnum<class "Retrieve and Visualize.lvclass">)
        n292 = Unbundle By Name(w659) -> ("IV"=w658:cluster{dbl[], dbl[]}[][][], "IV-2T"=w657:cluster{dbl[], dbl[]}[][][], "Vfast"=w666:dbl[][], "Vslow"=w665:dbl[], "Vslowest"=w664:dbl[], "Scan names"=w663:string[], "Comments"=→"Comments":string)
        n293 = Bundle By Name(cluster=w656, "3D.IV-4T"=w658, "3D.IV-2T"=w657, "Vfast"=w666, "Vslow"=w665, "Vslowest"=w664, "Scan Names"=w663) -> (w661:T15)
        n294 = call <vilib>:"Add State(s) to Queue__jki_lib_state_machine.vi"("State(s) in (\"\")"=w668) -> ("States Out"=w667:string)  [unwired: 14 in]
      }
      frame "Data Visualize: Index Config." {
        # "Template Separator\n(You can make a copy of, or modify, this frame)"
        n295 = Unbundle By Name(w671) -> ("R&V"=w670:refnum<class "Retrieve and Visualize.lvclass">)
        n296 = Unbundle By Name(w670) -> ("index"=w669:T2)
        n297 = local write "index"(w669) -> ()
        n298 = call <vilib>:"Add State(s) to Queue__jki_lib_state_machine.vi"("State(s) in (\"\")"=w674) -> ("States Out"=w673:string)  [unwired: 14 in]
      }
      frame "Data Visualize: Initialize Cursor Graph" {
        w679 = dbl[] []
        # "Initialize Cursor Graph"
        # "replace with array resize?"
        # "Do not put any code in this frame.\n(It is a separator no-op. You can make a copy of this frame to create a new UI frame)"
        n299 = Unbundle By Name(w675) -> ("Vfast"=w681:dbl[][], "Vslow"=w680:dbl[], "Scan Names"=w685:string[])
        n300 = Transpose 2D Array(2D array=w681) -> (transposed array=w676:dbl[][])
        n301 = for {
          tunnel: w676 -> [w694] mode=indexing
          tunnel: w680 -> [w691]
          shift-right: [w692] -> w682
          shift-left: w679 -> [w693]
          shift-right: [w690] -> w683
          shift-left: w679 -> [w689]
          n302 = Build Array (concatenate)(w693, w694) -> (w692:dbl[])
          n303 = Build Array (concatenate)(w689, w691) -> (w690:dbl[])
        }
        n304 = Index Array(array=w685) -> (element #1=w677:string, element #2=w684:string)  [unwired: 2 in]
        n305 = property on="Cursor Graph" class="XYGraph (strict)"("XScale.NameLbl.Text"=w677, "YScale.NameLbl.Text"=w684) -> ()  [unwired: 2 in, 2 out]
        n306 = Bundle(w682, w683) -> (→"Cursor Graph":cluster{dbl[], dbl[]})  [unwired: 1 in]
        n307 = call <vilib>:"Add State(s) to Queue__jki_lib_state_machine.vi"("State(s) in (\"\")"=w688) -> ("States Out"=w687:string)  [unwired: 14 in]
      }
      frame "Data Visualize: Subset" {
        # "IV-2T=I VS V2T"
        # "IV-4T=V4T VS V2T"
        # "Template Separator\n(You can make a copy of, or modify, this frame)"
        n308 = Unbundle By Name(w699) -> ("3D.IV-4T"=w702:cluster{dbl[], dbl[]}[][][], "3D.IV-2T"=w704:cluster{dbl[], dbl[]}[][][])
        n309 = for {
          tunnel: w702 -> [w712] mode=indexing
          tunnel: "Subset Slider (%) A" -> [w710]
          tunnel: [w709] -> w700 mode=indexing
          tunnel: w696 -> [w711]
          tunnel: [w708] -> w695
          n310 = for {
            tunnel: w712 -> [w713] mode=indexing
            tunnel: w710 -> [w718]
            tunnel: [w714] -> w709 mode=indexing
            tunnel: w711 -> [w717]
            tunnel: [w716] -> w708
            n311 = call-poly <userlib>:"Subset.vi"("error in (no error)"=w717, "Subset Method"=enum16{"Slider (%)", "X[] min and max"}."Slider (%)", "Subset Slider"=w718, "XY-data"=w713) -> ("error out"=w716:errorcluster, "Subset XY-data out"=w714:cluster{"X-array":dbl[], "Y-array":dbl[]}[])  [unwired: 6 in]
          }
        }
        n312 = for {
          tunnel: w704 -> [w723] mode=indexing
          tunnel: "Subset Slider (%) A" -> [w721]
          tunnel: [w720] -> w703 mode=indexing
          tunnel: w696 -> [w722]
          tunnel: [w719] -> w697
          n313 = for {
            tunnel: w723 -> [w727] mode=indexing
            tunnel: w721 -> [w729]
            tunnel: [w725] -> w720 mode=indexing
            tunnel: w722 -> [w728]
            tunnel: [w726] -> w719
            n314 = call-poly <userlib>:"Subset.vi"("error in (no error)"=w728, "Subset Method"=enum16{"Slider (%)", "X[] min and max"}."Slider (%)", "Subset Slider"=w729, "XY-data"=w727) -> ("error out"=w726:errorcluster, "Subset XY-data out"=w725:cluster{"X-array":dbl[], "Y-array":dbl[]}[])  [unwired: 6 in]
          }
        }
        n315 = Bundle By Name(cluster=w699, "3D.IV-4T"=w700, "3D.IV-2T"=w703) -> (w698:T15)
        n316 = Merge Errors(w695, w697) -> (w705:errorcluster)
        n317 = call <vilib>:"Add State(s) to Queue__jki_lib_state_machine.vi"("State(s) in (\"\")"=w707) -> ("States Out"=w706:string)  [unwired: 14 in]
      }
      frame "Data Visualize: Testing" {
        # "IV-2T=I VS V2T"
        # "IV-4T=V4T VS V2T"
        # "Template Separator\n(You can make a copy of, or modify, this frame)"
        n318 = Unbundle By Name(w732) -> ("3D.IV-4T"=w740:cluster{dbl[], dbl[]}[][][], "3D.IV-2T"=w738:cluster{dbl[], dbl[]}[][][])
        n319 = for {
          tunnel: w740 -> [w763] mode=indexing
          tunnel: [w761] -> w739 mode=indexing
          tunnel: w737 -> [w762]
          tunnel: [w760] -> w735
          tunnel: "averaging" -> [w759]
          tunnel: "decimating factor (1)" -> [w758]
          n320 = for {
            tunnel: w763 -> [w769] mode=indexing
            tunnel: [w768] -> w761 mode=indexing
            tunnel: w762 -> [w771]
            tunnel: [w767] -> w760
            tunnel: w759 -> [w765]
            tunnel: w758 -> [w764]
            # "sandbox"
            n321 = call-poly <userlib>:"Sort.vi"("error in (no error)"=w771, "XY-data"=w769) -> ("error out"=w770:errorcluster, "Sorted XY-data out"=w766:cluster{"X-array":dbl[], "Y-array":dbl[]}[])  [unwired: 7 in, 1 out]
            n322 = call-poly <userlib>:"Decimate.vi"("error in (no error)"=w770, "averaging (off)"=w765, "decimating factor (1)"=w764, "XY-data"=w766) -> ("error out"=w767:errorcluster, "Decimated XY-data out"=w768:cluster{"X-array":dbl[], "Y-array":dbl[]}[])  [unwired: 6 in]
          }
        }
        n323 = for {
          tunnel: w738 -> [w749] mode=indexing
          tunnel: [w747] -> w734 mode=indexing
          tunnel: w737 -> [w748]
          tunnel: [w746] -> w736
          tunnel: "decimating factor (1)" -> [w745]
          tunnel: "averaging" -> [w744]
          n324 = for {
            tunnel: w749 -> [w755] mode=indexing
            tunnel: [w754] -> w747 mode=indexing
            tunnel: w748 -> [w757]
            tunnel: [w753] -> w746
            tunnel: w745 -> [w751]
            tunnel: w744 -> [w750]
            n325 = call-poly <userlib>:"Sort.vi"("error in (no error)"=w757, "XY-data"=w755) -> ("error out"=w756:errorcluster, "Sorted XY-data out"=w752:cluster{"X-array":dbl[], "Y-array":dbl[]}[])  [unwired: 7 in, 1 out]
            n326 = call-poly <userlib>:"Decimate.vi"("error in (no error)"=w756, "averaging (off)"=w750, "decimating factor (1)"=w751, "XY-data"=w752) -> ("error out"=w753:errorcluster, "Decimated XY-data out"=w754:cluster{"X-array":dbl[], "Y-array":dbl[]}[])  [unwired: 6 in]
          }
        }
        n327 = Bundle By Name(cluster=w732, "3D.IV-4T"=w739, "3D.IV-2T"=w734) -> (w733:T15)
        n328 = Merge Errors(w735, w736) -> (w741:errorcluster)
        n329 = call <vilib>:"Add State(s) to Queue__jki_lib_state_machine.vi"("State(s) in (\"\")"=w743) -> ("States Out"=w742:string)  [unwired: 14 in]
      }
      frame "Data Visualize: SG Filter" {
        # "IV-2T=I VS V2T"
        # "IV-4T=V4T VS V2T"
        # "IV-2T=I VS V2T"
        # "IV-4T=V4T VS V2T"
        # "Template Separator\n(You can make a copy of, or modify, this frame)"
        n330 = Unbundle By Name(w773) -> ("3D.IV-4T"=w782:cluster{dbl[], dbl[]}[][][], "3D.IV-2T"=w778:cluster{dbl[], dbl[]}[][][])
        n331 = for {
          tunnel: [w800] -> w775 mode=indexing
          tunnel: "S-G side points (4T)" -> [w799]
          tunnel: w782 -> [w798] mode=indexing
          tunnel: w777 -> [w797]
          tunnel: [w796] -> w780
          n332 = for {
            tunnel: [w804] -> w800 mode=indexing
            tunnel: w799 -> [w805]
            tunnel: w798 -> [w803] mode=indexing
            tunnel: w797 -> [w802]
            tunnel: [w801] -> w796
            n333 = call-poly <userlib>:"Savitsky Golay Filter.vi"("error in (no error)"=w802, "side points"=w805, "XY-data"=w803) -> ("error out"=w801:errorcluster, "XY-data out"=w804:cluster{"X-array":dbl[], "Y-array":dbl[]}[])  [unwired: 7 in]
          }
        }
        n334 = for {
          tunnel: [w790] -> w776 mode=indexing
          tunnel: w778 -> [w789] mode=indexing
          tunnel: "S-G side points (2T)" -> [w786]
          tunnel: w777 -> [w788]
          tunnel: [w787] -> w781
          n335 = for {
            tunnel: [w795] -> w790 mode=indexing
            tunnel: w789 -> [w794] mode=indexing
            tunnel: w786 -> [w791]
            tunnel: w788 -> [w793]
            tunnel: [w792] -> w787
            n336 = call-poly <userlib>:"Savitsky Golay Filter.vi"("error in (no error)"=w793, "side points"=w791, "XY-data"=w794) -> ("error out"=w792:errorcluster, "XY-data out"=w795:cluster{"X-array":dbl[], "Y-array":dbl[]}[])  [unwired: 7 in]
          }
        }
        n337 = Bundle By Name(cluster=w773, "3D.IV-4T"=w775, "3D.IV-2T"=w776) -> (w772:T15)
        n338 = Merge Errors(w780, w781) -> (w783:errorcluster)
        n339 = call <vilib>:"Add State(s) to Queue__jki_lib_state_machine.vi"("State(s) in (\"\")"=w785) -> ("States Out"=w784:string)  [unwired: 14 in]
      }
      frame "Data Visualize: Calculate Derivative 2T" {
        w815 = enum16{"y/x vs x", "x/y vs y"}."y/x vs x" ("Type 2")
        # "IV-2T=I VS V2T"
        # "IV-4T=V4T VS V2T"
        # "dV2T/dI vs I"
        # "dI/dV2T vs V2T"
        # "dV4T/dV2T vs V2T"
        # "Template Separator\n(You can make a copy of, or modify, this frame)"
        n340 = local read "Window [h]"() -> (w806:dbl)
        n341 = Unbundle By Name(w809) -> ("3D.IV-4T"=w818:cluster{dbl[], dbl[]}[][][], "3D.IV-2T"=w817:cluster{dbl[], dbl[]}[][][])
        n342 = for {
          tunnel: w817 -> [w827] mode=indexing
          tunnel: [w825] -> w811 mode=indexing
          tunnel: w815 -> [w823]
          tunnel: w806 -> [w822]
          tunnel: enum16{"y/x vs x", "x/y vs y"}."x/y vs y" ("Type 2") -> [w820]
          tunnel: [w821] -> w812 mode=indexing
          tunnel: w808 -> [w826]
          tunnel: [w824] -> w816
          n343 = for {
            tunnel: w827 -> [w837] mode=indexing
            tunnel: [w831] -> w825 mode=indexing
            tunnel: w823 -> [w829]
            tunnel: w822 -> [w830]
            tunnel: w820 -> [w828]
            tunnel: [w832] -> w821 mode=indexing
            tunnel: w826 -> [w836]
            tunnel: [w833] -> w824
            n344 = call-poly <userlib>:"Difference Quotient.vi"("error in (no error)"=w836, "Type"=w829, "Window [h] (2)"=w830, "XY-data"=w837) -> ("error out"=w834:errorcluster, "Difference Quotient"=w831:cluster{"X-array":dbl[], "Y-array":dbl[]}[], "XY-data out"=w835:cluster{"X-array":dbl[], "Y-array":dbl[]}[])  [unwired: 5 in]
            n345 = call-poly <userlib>:"Difference Quotient.vi"("error in (no error)"=w834, "Type"=w828, "Window [h] (2)"=w830, "XY-data"=w835) -> ("error out"=w833:errorcluster, "Difference Quotient"=w832:cluster{"X-array":dbl[], "Y-array":dbl[]}[])  [unwired: 5 in, 1 out]
          }
        }
        n346 = for {
          tunnel: w818 -> [w843] mode=indexing
          tunnel: [w841] -> w810 mode=indexing
          tunnel: w815 -> [w839]
          tunnel: w806 -> [w838]
          tunnel: w808 -> [w842]
          tunnel: [w840] -> _
          n347 = for {
            tunnel: w843 -> [w849] mode=indexing
            tunnel: [w847] -> w841 mode=indexing
            tunnel: w839 -> [w844]
            tunnel: w838 -> [w845]
            tunnel: w842 -> [w848]
            tunnel: [w846] -> w840
            n348 = call-poly <userlib>:"Difference Quotient.vi"("error in (no error)"=w848, "Type"=w844, "Window [h] (2)"=w845, "XY-data"=w849) -> ("error out"=w846:errorcluster, "Difference Quotient"=w847:cluster{"X-array":dbl[], "Y-array":dbl[]}[])  [unwired: 5 in, 1 out]
          }
        }
        n349 = Bundle By Name(cluster=w809, "3D.G-4T"=w810, "3D.R-4T"=w810, "3D.G-2T"=w811, "3D.R-2T"=w812) -> (w813:T15)
        n350 = call <vilib>:"Add State(s) to Queue__jki_lib_state_machine.vi"("State(s) in (\"\")"=w814) -> ("States Out"=w819:string)  [unwired: 14 in]
      }
      frame "Data Visualize: Calculate Derivative 4T" {
        # "Template Separator\n(You can make a copy of, or modify, this frame)"
        n351 = Unbundle By Name(w851) -> ("3D.R-2T"=w858:cluster{dbl[], dbl[]}[][][], "3D.R-4T"=w855:cluster{dbl[], dbl[]}[][][], "3D.IV-4T"=w854:cluster{dbl[], dbl[]}[][][])
        n352 = for {
          tunnel: w858 -> [w864] mode=indexing
          tunnel: w855 -> [w863] mode=indexing
          tunnel: w854 -> [w862] mode=indexing
          tunnel: [w861] -> w853 mode=indexing
          tunnel: [w860] -> w852 mode=indexing
          n353 = for {
            tunnel: w864 -> [w869] mode=indexing
            tunnel: w863 -> [w868] mode=indexing
            tunnel: w862 -> [w867] mode=indexing
            tunnel: [w866] -> w861 mode=indexing
            tunnel: [w865] -> w860 mode=indexing
            n354 = for {
              tunnel: w869 -> [w884] mode=indexing
              tunnel: w868 -> [w883] mode=indexing
              tunnel: w867 -> [w882] mode=indexing
              tunnel: [w870] -> w866 mode=indexing
              tunnel: [w881] -> w865 mode=indexing
              # "R4T =dV4T/dV2T vs V2T"
              # "R2T =dV2T/dI vs I"
              # "V4T vs V2T"
              n355 = Unbundle(w882) -> (w873:dbl[])  [unwired: 1 out]
              n356 = Unbundle(w883) -> (w877:dbl[])  [unwired: 1 out]
              n357 = Unbundle(w884) -> (w880:dbl[], w878:dbl[])
              n358 = Multiply(x=w878, y=w877) -> (x*y=w876:dbl[])
              n359 = Reciprocal(x=w876) -> (1/x=w872:dbl[])
              n360 = call "Remove NaNs.vi"("Array in"=w880) -> ("Array out"=w879:dbl[])
              n361 = call "Remove NaNs.vi"("Array in"=w876) -> ("Array out"=w875:dbl[])
              n362 = call "Remove NaNs.vi"("Array in"=w872) -> ("Array out"=w871:dbl[])
              n363 = call "Remove NaNs.vi"("Array in"=w873) -> ("Array out"=w874:dbl[])
              n364 = Bundle("Array out"=w879, "Array out"=w875) -> (w870:cluster{"Array out":dbl[], "Array out":dbl[]})  [unwired: 1 in]
              n365 = Bundle("Array out"=w874, "Array out"=w871) -> (w881:cluster{"Array out":dbl[], "Array out":dbl[]})  [unwired: 1 in]
            }
          }
        }
        n366 = Bundle By Name(cluster=w851, "3D.R-4T"=w853, "3D.G-4T"=w852) -> (w856:T15)
        n367 = call <vilib>:"Add State(s) to Queue__jki_lib_state_machine.vi"("State(s) in (\"\")"=w857) -> ("States Out"=w859:string)  [unwired: 14 in]
      }
      frame "Data Visualize: Calculate Transconductance" {
        # "Template Separator\n(You can make a copy of, or modify, this frame)"
        n368 = Unbundle By Name(w891) -> ("Vfast Slice"=w888:dbl[], "3D.G-4T"=w889:cluster{dbl[], dbl[]}[][][])
        n369 = for {
          tunnel: w889 -> [w898] mode=indexing
          tunnel: w888 -> [w896]
          tunnel: w885 -> [w897]
          tunnel: [w895] -> w887 mode=indexing
          tunnel: [w894] -> w886
          n370 = for {
            tunnel: w898 -> [w909] mode=indexing
            tunnel: w897 -> [w907]
            tunnel: w896 -> [w906]
            tunnel: [w903] -> w895 mode=indexing
            tunnel: [w901] -> w894
            n371 = local read "Transconductance [h]"() -> (w899:dbl)
            n372 = call <userlib>:"XY to 2D.vi"("error in (no error)"=w907, "XY-data"=w909) -> ("error out"=w905:errorcluster, "X Array"=w900:dbl[], "2D Y Array"=w908:dbl[][])  [unwired: 6 in, 1 out]
            n373 = call "Derivative (2D).vi"("error in (no error)"=w905, "Window [h] (2)"=w899, "Axis Array"=w906, "Conductance"=w908) -> ("error out"=w902:errorcluster, "Transconductance"=w904:dbl[][])  [unwired: 5 in, 1 out]
            n374 = call <userlib>:"2D to XY.vi"("error in (no error)"=w902, "X Array"=w900, "2D Y Array"=w904) -> ("error out"=w901:errorcluster, "XY-data out"=w903:cluster{"X-array":dbl[], "Y-array":dbl[]}[])  [unwired: 7 in]
          }
        }
        n375 = Bundle By Name(cluster=w891, "3D.dG-4T"=w887) -> (w890:T15)
        n376 = call <vilib>:"Add State(s) to Queue__jki_lib_state_machine.vi"("State(s) in (\"\")"=w893) -> ("States Out"=w892:string)  [unwired: 14 in]
      }
      frame "Data Visualize: IV 4T IV 2T" {
        # "V2 vs I"
        # "V4 vs I"
        # "I VS V2T"
        # "V4T VS V2T"
        # "Template Separator\n(You can make a copy of, or modify, this frame)"
        n377 = Unbundle By Name(w911) -> ("3D.IV-4T"=w916:cluster{dbl[], dbl[]}[][][], "3D.IV-2T"=w915:cluster{dbl[], dbl[]}[][][])
        n378 = for {
          tunnel: w916 -> [w922] mode=indexing
          tunnel: w915 -> [w921] mode=indexing
          tunnel: [w920] -> w914 mode=indexing
          tunnel: [w919] -> w913 mode=indexing
          n379 = for {
            tunnel: w922 -> [w926] mode=indexing
            tunnel: w921 -> [w925] mode=indexing
            tunnel: [w924] -> w920 mode=indexing
            tunnel: [w923] -> w919 mode=indexing
            n380 = for {
              tunnel: w926 -> [w933] mode=indexing
              tunnel: w925 -> [w932] mode=indexing
              tunnel: [w931] -> w924 mode=indexing
              tunnel: [w930] -> w923 mode=indexing
              n381 = Unbundle(w933) -> (w929:dbl[])  [unwired: 1 out]
              n382 = Unbundle(w932) -> (w927:dbl[], w928:dbl[])
              n383 = Bundle(w928, w929) -> (w931:cluster{dbl[], dbl[]})  [unwired: 1 in]
              n384 = Bundle(w928, w927) -> (w930:cluster{dbl[], dbl[]})  [unwired: 1 in]
            }
          }
        }
        n385 = Bundle By Name(cluster=w911, "3D.IV-4T"=w914, "3D.IV-2T"=w913) -> (w910:T15)
        n386 = call <vilib>:"Add State(s) to Queue__jki_lib_state_machine.vi"("State(s) in (\"\")"=w918) -> ("States Out"=w917:string)  [unwired: 14 in]
      }
      frame "Data Visualize: Calculate Indices" {
        # "used?"
        # "used?"
        # "used?"
        # "Calculate Indices"
        # "Template Separator\n(You can make a copy of, or modify, this frame)"
        n387 = Unbundle By Name(w935) -> ("Vfast"=w948:dbl[][], "Vslow"=w934:dbl[], "Vslowest"=w947:dbl[])
        n388 = property on="Cursor Graph" class="XYGraph (strict)"(error in=w943) -> (error out=w937:errorcluster, "Cursor.Cursor X"=w938:dbl, "Cursor.Cursor Y"=w939:dbl)  [unwired: 1 in, 1 out]
        "Slow" <- w939
        "Fast" <- w938
        n389 = Index Array(array=w947, index="Field/Temperature") -> (element=→"slowest":dbl)
        n390 = call "Calculate Indices.vi"("Cursor.Cursor Y"=w939, "Cursor.Cursor X"=w938, "Vslow"=w934, "Vfast"=w948) -> ("Column"=w941:i32, "Row"=w944:i32, "Column Array"=w945:i32[], "Row Array"=w936:i32[])  [unwired: 4 in]
        n391 = Array Size(array=w947) -> (size(s)=w949:i32)
        n392 = Decrement(x=w949) -> (x-1=w950:i32)
        n393 = Index Array(array=w948, index (row)=w944) -> (element=w946:dbl[])  [unwired: 1 in]
        n394 = property on="Field/Temperature" class="Slide (strict)"("Scale.Maximum"=w950) -> ()  [unwired: 2 in, 2 out]
        n395 = Bundle By Name(cluster=w935, "Vfast Slice"=w946, "Vslow Slice"=w934, "Page"="Field/Temperature", "Row []"=w936, "Column []"=w945, "Row"=w944, "Column"=w941) -> (w942:T15)
        n396 = call <vilib>:"Add State(s) to Queue__jki_lib_state_machine.vi"("State(s) in (\"\")"=w953) -> ("States Out"=w952:string)  [unwired: 14 in]
      }
      frame "Data Visualize: XY Graphs" {
        # "Template Separator\n(You can make a copy of, or modify, this frame)"
        n397 = Unbundle By Name(w955) -> ("3D"=w962:T17)
        n398 = Unbundle By Name(w962) -> ("IV-4T"=w968:cluster{dbl[], dbl[]}[][][], "IV-2T"=w967:cluster{dbl[], dbl[]}[][][], "G-4T"=w966:cluster{dbl[], dbl[]}[][][], "R-4T"=w965:cluster{dbl[], dbl[]}[][][], "G-2T"=w964:cluster{dbl[], dbl[]}[][][], "R-2T"=w963:cluster{dbl[], dbl[]}[][][])
        n399 = case shown="\"Vary Fields\"" "XY Data" {
          tunnel: w968 -> [w986 w1001 w1016]
          tunnel: w967 -> [w985 w1000 w1015]
          tunnel: w966 -> [w984 w999 w1014]
          tunnel: w965 -> [w983 w998 w1013]
          tunnel: w964 -> [w982 w997 w1012]
          tunnel: w963 -> [w981 w996 w1011]
          tunnel: [w980 w995 w1010] -> w961
          tunnel: [w979 w994 w1009] -> w960
          tunnel: [w978 w993 w1008] -> w959
          tunnel: [w977 w992 w1007] -> w958
          tunnel: [w976 w991 w1006] -> w957
          tunnel: [w973 w990 w1005] -> w956
          tunnel: w955 -> [w974 w989 w1003]
          frame "Vary Vfast" {
            # "row"
            # "page"
            n400 = Unbundle By Name(w974) -> ("Row"=w975:i32, "Column"=w972:i32)
            n401 = Index Array(array=w986, index (dim 0)=w975, index (dim 2)=w972) -> (element=w980:cluster{dbl[], dbl[]}[])  [unwired: 1 in]
            n402 = Index Array(array=w985, index (dim 0)=w975, index (dim 2)=w972) -> (element=w979:cluster{dbl[], dbl[]}[])  [unwired: 1 in]
            n403 = Index Array(array=w984, index (dim 0)=w975, index (dim 2)=w972) -> (element=w978:cluster{dbl[], dbl[]}[])  [unwired: 1 in]
            n404 = Index Array(array=w983, index (dim 0)=w975, index (dim 2)=w972) -> (element=w977:cluster{dbl[], dbl[]}[])  [unwired: 1 in]
            n405 = Index Array(array=w982, index (dim 0)=w975, index (dim 2)=w972) -> (element=w976:cluster{dbl[], dbl[]}[])  [unwired: 1 in]
            n406 = Index Array(array=w981, index (dim 0)=w975, index (dim 2)=w972) -> (element=w973:cluster{dbl[], dbl[]}[])  [unwired: 1 in]
          }
          frame "Vary Vslow" {
            n407 = Unbundle By Name(w989) -> ("Row"=w987:i32, "Column"=w988:i32)
            n408 = Index Array(array=w1001, index (dim 0)=w987, index (dim 1)=w988) -> (element=w995:cluster{dbl[], dbl[]}[])  [unwired: 1 in]
            n409 = Index Array(array=w1000, index (dim 0)=w987, index (dim 1)=w988) -> (element=w994:cluster{dbl[], dbl[]}[])  [unwired: 1 in]
            n410 = Index Array(array=w999, index (dim 0)=w987, index (dim 1)=w988) -> (element=w993:cluster{dbl[], dbl[]}[])  [unwired: 1 in]
            n411 = Index Array(array=w998, index (dim 0)=w987, index (dim 1)=w988) -> (element=w992:cluster{dbl[], dbl[]}[])  [unwired: 1 in]
            n412 = Index Array(array=w997, index (dim 0)=w987, index (dim 1)=w988) -> (element=w991:cluster{dbl[], dbl[]}[])  [unwired: 1 in]
            n413 = Index Array(array=w996, index (dim 0)=w987, index (dim 1)=w988) -> (element=w990:cluster{dbl[], dbl[]}[])  [unwired: 1 in]
          }
          frame "Vary Fields" {
            # "column"
            # "row"
            n414 = Unbundle By Name(w1003) -> ("Row"=w1004:i32, "Column"=w1002:i32)
            n415 = Index Array(array=w1016, index (dim 1)=w1004, index (dim 2)=w1002) -> (element=w1010:cluster{dbl[], dbl[]}[])  [unwired: 1 in]
            n416 = Index Array(array=w1015, index (dim 1)=w1004, index (dim 2)=w1002) -> (element=w1009:cluster{dbl[], dbl[]}[])  [unwired: 1 in]
            n417 = Index Array(array=w1014, index (dim 1)=w1004, index (dim 2)=w1002) -> (element=w1008:cluster{dbl[], dbl[]}[])  [unwired: 1 in]
            n418 = Index Array(array=w1013, index (dim 1)=w1004, index (dim 2)=w1002) -> (element=w1007:cluster{dbl[], dbl[]}[])  [unwired: 1 in]
            n419 = Index Array(array=w1012, index (dim 1)=w1004, index (dim 2)=w1002) -> (element=w1006:cluster{dbl[], dbl[]}[])  [unwired: 1 in]
            n420 = Index Array(array=w1011, index (dim 1)=w1004, index (dim 2)=w1002) -> (element=w1005:cluster{dbl[], dbl[]}[])  [unwired: 1 in]
          }
        }
        "IV 4T" <- w961
        "dI/dV (G)" <- w959
        "IV 2T" <- w960
        "dI/dV (G) 2T" <- w957
        "dV/dI (R)" <- w958
        "dV/dI (R) 2T" <- w956
        n421 = call <vilib>:"Add State(s) to Queue__jki_lib_state_machine.vi"("State(s) in (\"\")"=w971) -> ("States Out"=w970:string)  [unwired: 14 in]
      }
      frame "Data Visualize: Choose Data 1" {
        # "Slice at constant B"
        # "Template Separator\n(You can make a copy of, or modify, this frame)"
        n422 = local read "Intensity 1"() -> (w1018:T7)
        n423 = Unbundle By Name(w1043) -> ("Vfast Slice"=w1020:dbl[], "Graph.Intensity 1"=w1041:refnum<class "graph_utilities.lvclass">, "3D"=w1042:T17, "Row"=w1035:i32, "Page"=w1017:i32)
        n424 = local read "Transconductance [h]"() -> (w1019:dbl)
        n425 = case shown="\"dGdVsg-4T\"" w1018 {
          tunnel: w1042 -> [w1055 w1057 w1059 w1061 w1063 w1065 w1067 w1069]
          tunnel: [w1054 w1056 w1058 w1060 w1062 w1064 w1066 w1068] -> w1028
          frame "IV-4T", Default {
            n426 = Unbundle By Name(w1055) -> ("IV-4T"=w1054:cluster{dbl[], dbl[]}[][][])
          }
          frame "IV-2T" {
            n427 = Unbundle By Name(w1057) -> ("IV-2T"=w1056:cluster{dbl[], dbl[]}[][][])
          }
          frame "R-4T" {
            n428 = Unbundle By Name(w1059) -> ("R-4T"=w1058:cluster{dbl[], dbl[]}[][][])
          }
          frame "G-4T" {
            n429 = Unbundle By Name(w1061) -> ("G-4T"=w1060:cluster{dbl[], dbl[]}[][][])
          }
          frame "R-2T" {
            n430 = Unbundle By Name(w1063) -> ("R-2T"=w1062:cluster{dbl[], dbl[]}[][][])
          }
          frame "G-2T" {
            n431 = Unbundle By Name(w1065) -> ("G-2T"=w1064:cluster{dbl[], dbl[]}[][][])
          }
          frame "dGdVsg-4T" {
            n432 = Unbundle By Name(w1067) -> ("G-4T"=w1066:cluster{dbl[], dbl[]}[][][])
          }
          frame "dGdVsg-2T" {
            n433 = Unbundle By Name(w1069) -> ("G-2T"=w1068:cluster{dbl[], dbl[]}[][][])
          }
        }
        n434 = Index Array(array=w1028, index (dim 0)=w1035, index (dim 2)=w1017) -> (element=w1025:cluster{dbl[], dbl[]}[])  [unwired: 1 in]
        n435 = call <userlib>:"XY to 2D.vi"("error in (no error)"=w1026, "Fake Point"="fake point 1", "Interpolate [T]"=TRUE, "XY-data"=w1025) -> ("error out"=w1031:errorcluster, "X Array"=w1029:dbl[], "2D Y Array"=w1030:dbl[][])  [unwired: 4 in, 1 out]
        n436 = call "G to e2h (2D).vi"("error in (no error)"=w1031, "e^2/h?"="e^2/h? 1", "Array in"=w1030) -> ("error out"=w1034:errorcluster, "Array out"=w1040:dbl[][])  [unwired: 7 in]
        n437 = call "Log (2D).vi"("error in (no error)"=w1034, "Log scale?"="Log scale? 1", "Array in"=w1040) -> ("error out"=w1021:errorcluster, "Array out"=w1024:dbl[][])  [unwired: 7 in]
        n438 = case shown="\"dGdVsg-4T\", \"dGdVsg-2T\"" w1018 {
          tunnel: w1021 -> [w1047 w1053]
          tunnel: w1024 -> [w1046 w1052]
          tunnel: [w1046 w1051] -> w1023
          tunnel: [w1047 w1050] -> w1022
          tunnel: w1020 -> [_ w1049]
          tunnel: w1019 -> [_ w1048]
          frame Default {
          }
          frame "dGdVsg-4T", "dGdVsg-2T" {
            n439 = call "Derivative (2D).vi"("error in (no error)"=w1053, "Window [h] (2)"=w1048, "Axis Array"=w1049, "Conductance"=w1052) -> ("error out"=w1050:errorcluster, "Transconductance"=w1051:dbl[][])  [unwired: 5 in, 1 out]
          }
        }
        "Intensity Graph 1" <- w1023
        n440 = Subtract(x=w1029, y="X Offset 1") -> (x-y=w1036:dbl[])
        n441 = call <userlib>:"Set Intensity Graph X Scale Array.vi"("error in (no error)"=w1022, "X Scale"=w1036, "graph_utilities in"=w1041) -> ("error out"=w1038:errorcluster)  [unwired: 7 in, 1 out]
        n442 = call <vilib>:"Add State(s) to Queue__jki_lib_state_machine.vi"("State(s) in (\"\")"=w1045) -> ("States Out"=w1044:string)  [unwired: 14 in]
      }
      frame "Data Visualize: Choose Data 2" {
        # "Template Separator\n(You can make a copy of, or modify, this frame)"
        n443 = Unbundle By Name(w1082) -> ("Vfast Slice"=w1072:dbl[], "Graph.Intensity 2"=w1095:refnum<class "graph_utilities.lvclass">, "3D"=w1096:T17, "Row"=w1087:i32, "Page"=w1071:i32)
        n444 = local read "Intensity 2"() -> (w1073:T7)
        n445 = case shown="\"dGdVsg-2T\"" w1073 {
          tunnel: w1096 -> [w1108 w1110 w1112 w1114 w1116 w1118 w1120 w1122]
          tunnel: [w1107 w1109 w1111 w1113 w1115 w1117 w1119 w1121] -> w1088
          frame "IV-4T", Default {
            n446 = Unbundle By Name(w1108) -> ("IV-4T"=w1107:cluster{dbl[], dbl[]}[][][])
          }
          frame "IV-2T" {
            n447 = Unbundle By Name(w1110) -> ("IV-2T"=w1109:cluster{dbl[], dbl[]}[][][])
          }
          frame "R-4T" {
            n448 = Unbundle By Name(w1112) -> ("R-4T"=w1111:cluster{dbl[], dbl[]}[][][])
          }
          frame "G-4T" {
            n449 = Unbundle By Name(w1114) -> ("G-4T"=w1113:cluster{dbl[], dbl[]}[][][])
          }
          frame "R-2T" {
            n450 = Unbundle By Name(w1116) -> ("R-2T"=w1115:cluster{dbl[], dbl[]}[][][])
          }
          frame "G-2T" {
            n451 = Unbundle By Name(w1118) -> ("G-2T"=w1117:cluster{dbl[], dbl[]}[][][])
          }
          frame "dGdVsg-4T" {
            n452 = Unbundle By Name(w1120) -> ("G-4T"=w1119:cluster{dbl[], dbl[]}[][][])
          }
          frame "dGdVsg-2T" {
            n453 = Unbundle By Name(w1122) -> ("G-2T"=w1121:cluster{dbl[], dbl[]}[][][])
          }
        }
        n454 = Index Array(array=w1088, index (dim 0)=w1087, index (dim 2)=w1071) -> (element=w1078:cluster{dbl[], dbl[]}[])  [unwired: 1 in]
        n455 = call <userlib>:"XY to 2D.vi"("error in (no error)"=w1079, "Fake Point"="fake point 2", "Interpolate [T]"=TRUE, "XY-data"=w1078) -> ("error out"=w1083:errorcluster, "X Array"=w1085:dbl[], "2D Y Array"=w1081:dbl[][])  [unwired: 4 in, 1 out]
        n456 = local read "Transconductance [h]"() -> (w1070:dbl)
        n457 = call "G to e2h (2D).vi"("error in (no error)"=w1083, "e^2/h?"="e^2/h? 2", "Array in"=w1081) -> ("error out"=w1093:errorcluster, "Array out"=w1094:dbl[][])  [unwired: 7 in]
        n458 = Subtract(x=w1085, y="X Offset 2") -> (x-y=w1090:dbl[])
        n459 = call "Log (2D).vi"("error in (no error)"=w1093, "Log scale?"="Log scale? 2", "Array in"=w1094) -> ("error out"=w1077:errorcluster, "Array out"=w1076:dbl[][])  [unwired: 7 in]
        n460 = case shown="Default" w1073 {
          tunnel: w1077 -> [w1100 w1106]
          tunnel: w1076 -> [w1099 w1105]
          tunnel: [w1099 w1104] -> w1075
          tunnel: [w1100 w1103] -> w1074
          tunnel: w1072 -> [_ w1102]
          tunnel: w1070 -> [_ w1101]
          frame Default {
          }
          frame "dGdVsg-4T", "dGdVsg-2T" {
            n461 = call "Derivative (2D).vi"("error in (no error)"=w1106, "Window [h] (2)"=w1101, "Axis Array"=w1102, "Conductance"=w1105) -> ("error out"=w1103:errorcluster, "Transconductance"=w1104:dbl[][])  [unwired: 5 in, 1 out]
          }
        }
        "Intensity Graph 2" <- w1075
        n462 = call <userlib>:"Set Intensity Graph X Scale Array.vi"("error in (no error)"=w1074, "X Scale"=w1090, "graph_utilities in"=w1095) -> ("error out"=w1091:errorcluster)  [unwired: 7 in, 1 out]
        n463 = call <vilib>:"Add State(s) to Queue__jki_lib_state_machine.vi"("State(s) in (\"\")"=w1098) -> ("States Out"=w1097:string)  [unwired: 14 in]
      }
      frame "Data Visualize: 3D" {
        w1130 = 0 ("index (vol)")
        # "X gate vs Y gate"
        # "X gate vs I"
        # "Y gate vs I"
        # "Vfast"
        # "Vslow"
        # "Vfastest"
        # "convert 3D XY cluster to 4D array"
        # "Template Separator\n(You can make a copy of, or modify, this frame)"
        n464 = local read "Intensity 3D"() -> (w1141:T7)
        n465 = Unbundle By Name(w1132) -> ("Vslow"=w1142:dbl[], "Vfast"=w1143:dbl[][], "3D"=w1138:T17, "Row"=w1134:i32)  [unwired: 1 out]
        n466 = case shown="\"dGdVsg-4T\"" w1141 {
          tunnel: w1138 -> [w1158 w1160 w1162 w1164 w1166 w1168 w1170]
          tunnel: [w1157 w1159 w1161 w1163 w1165 w1167 w1169] -> w1137
          frame "IV-4T", Default {
            n467 = Unbundle By Name(w1158) -> ("IV-4T"=w1157:cluster{dbl[], dbl[]}[][][])
          }
          frame "IV-2T" {
            n468 = Unbundle By Name(w1160) -> ("IV-2T"=w1159:cluster{dbl[], dbl[]}[][][])
          }
          frame "R-4T" {
            n469 = Unbundle By Name(w1162) -> ("R-4T"=w1161:cluster{dbl[], dbl[]}[][][])
          }
          frame "G-4T" {
            n470 = Unbundle By Name(w1164) -> ("G-4T"=w1163:cluster{dbl[], dbl[]}[][][])
          }
          frame "R-2T" {
            n471 = Unbundle By Name(w1166) -> ("R-2T"=w1165:cluster{dbl[], dbl[]}[][][])
          }
          frame "G-2T" {
            n472 = Unbundle By Name(w1168) -> ("G-2T"=w1167:cluster{dbl[], dbl[]}[][][])
          }
          frame "dGdVsg-4T" {
            n473 = Unbundle By Name(w1170) -> ("G-4T"=w1169:cluster{dbl[], dbl[]}[][][])
          }
        }
        n474 = for {
          tunnel: w1137 -> [w1151] mode=indexing
          tunnel: [w1150] -> w1135 mode=indexing
          tunnel: [w1149] -> w1125 mode=indexing
          n475 = for {
            tunnel: w1151 -> [w1156] mode=indexing
            tunnel: [w1155] -> w1149 mode=indexing
            tunnel: [w1153] -> w1150 mode=indexing
            tunnel: [w1152] -> _ mode=indexing
            n476 = call <userlib>:"XY to 2D.vi"("Interpolate [T]"=TRUE, "XY-data"=w1156) -> ("error out"=w1152:errorcluster, "X Array"=w1153:dbl[], "2D Y Array"=w1155:dbl[][])  [unwired: 6 in, 1 out]
          }
        }
        n477 = Index Array(array=w1143) -> (element=w1140:dbl[])  [unwired: 2 in]
        n478 = property on="x3D Graph 9" class="IntGraph (strict)"() -> ("Cursor.Cursor Index"=w1131:i32, "Cursor.Cursor Plot"=w1126:i32)  [unwired: 2 in, 2 out]
        n479 = Index Array(array=w1135, index (dim 0)=0 ("disabled index (page)"), index (dim 1)=w1134) -> (element=w1123:dbl[])  [unwired: 1 in]
        n480 = call <userlib>:"Array to Offset and Multiplier.vi"("Array"=w1142) -> ("Offset and Multiplier"=w1139:T11)
        n481 = call <userlib>:"Array to Offset and Multiplier.vi"("Array"=w1140) -> ("Offset and Multiplier"=w1133:T11)
        n482 = property on="x3D Graph 10" class="IntGraph (strict)"("Cursor.Cursor Plot"=w1126) -> ("Cursor.Cursor Index"=w1146:i32)  [unwired: 2 in, 2 out]
        n483 = call <userlib>:"Array to Offset and Multiplier.vi"("Array"=w1123) -> ("Offset and Multiplier"=w1136:T11)
        n484 = property on="x3D Graph 9" class="IntGraph (strict)"("XScale.Ofst&Mult"=w1136, "YScale.Ofst&Mult"=w1139) -> ()  [unwired: 2 in, 2 out]
        n485 = property on="x3D Graph 10" class="IntGraph (strict)"("XScale.Ofst&Mult"=w1133, "YScale.Ofst&Mult"=w1139) -> ()  [unwired: 2 in, 2 out]
        n486 = property on="x3D Graph 11" class="IntGraph (strict)"("XScale.Ofst&Mult"=w1136, "YScale.Ofst&Mult"=w1133) -> ()  [unwired: 2 in, 2 out]
        n487 = Index Array(array=w1125, index (dim 0) #1=w1130, index (dim 1) #1=w1146, index (dim 0) #2=w1130, index (dim 2) #2=w1131, index (dim 0) #3=w1130, index (dim 3) #3=w1126) -> (element #1=→"x3D Graph 9":dbl[][], element #2=→"x3D Graph 10":dbl[][], element #3=w1128:dbl[][])  [unwired: 6 in]
        n488 = Transpose 2D Array(2D array=w1128) -> (transposed array=→"x3D Graph 11":dbl[][])
        n489 = call <vilib>:"Add State(s) to Queue__jki_lib_state_machine.vi"("State(s) in (\"\")"=w1148) -> ("States Out"=w1147:string)  [unwired: 14 in]
      }
      frame "---------- Data Export ----------" {
        # "Template Separator\n(You can make a copy of, or modify, this frame)"
        n490 = call <vilib>:"Add State(s) to Queue__jki_lib_state_machine.vi"("State(s) in (\"\")"=w1174) -> ("States Out"=w1173:string)  [unwired: 14 in]
      }
      frame "Data Export: Export" {
        # "Template Separator\n(You can make a copy of, or modify, this frame)"
        n491 = Unbundle By Name(w1175) -> ("Graph"=w1181:T16)
        n492 = case shown="\"V Cut 2\"" "Export What?" {
          selector: "Export What?" -> [w1184 w1199 w1215 w1231 w1250 w1269]
          tunnel: w1181 -> [w1196 w1213 w1230 w1243 w1260 w1277]
          tunnel: w1178 -> [w1193 w1203 w1222 w1239 w1246 w1262]
          tunnel: [w1191 w1210 w1227 w1238 w1257 w1274] -> w1180
          tunnel: "Export ITX Path" -> [w1188 w1201 w1218 w1233 w1256 w1268]
          tunnel: "Export ITX Name" -> [w1187 w1202 w1217 w1234 w1252 w1271]
          frame "Intensity 1", Default {
            n493 = local read "Intensity 1"() -> (w1185:T7)
            n494 = Format Into String(format string="%s-%s-%s-", w1187, w1185, w1184) -> (resulting string=w1190:string)  [unwired: 2 in, 1 out]
            n495 = Unbundle By Name(w1196) -> ("Intensity 1"=w1195:refnum<class "graph_utilities.lvclass">)
            n496 = Build Path(base path=w1188, name or relative path=w1190) -> (appended path=w1186:path)
            n497 = call <userlib>:"Read Intensity Graph ref.vi"("error in (no error)"=w1193, "graph_utilities in"=w1195) -> ("error out"=w1192:errorcluster, "Intensity Graph"=w1194:refnum<vi>)  [unwired: 6 in, 2 out]
            n498 = call <userlib>:"Intensity Graph to Igor Graph.vi"("error in (no error)"=w1192, "Intensity Graph Reference"=w1194, "Path"=w1186) -> ("error out"=w1191:errorcluster)  [unwired: 7 in, 1 out]
          }
          frame "H Cut 1" {
            n499 = local read "Intensity 1"() -> (w1198:T7)
            n500 = Unbundle By Name(w1213) -> ("H 1"=w1206:refnum<class "graph_utilities.lvclass">)
            n501 = call <userlib>:"Get Intensity Graph Cursor (Control).vi"("error in (no error)"=w1203, "graph_utilities in"=w1206) -> ("error out"=w1204:errorcluster, "Cursor.Cursor Position"=w1207:T20, "graph_utilities out"=w1205:refnum<class "graph_utilities.lvclass">)  [unwired: 7 in]
            n502 = Unbundle By Name(w1207) -> ("Y"=w1200:dbl)
            n503 = Format Into String(format string="%s-%s-%s-%f-", w1202, w1198, w1199, w1200) -> (resulting string=w1209:string)  [unwired: 2 in, 1 out]
            n504 = call <userlib>:"Read XY Graph ref.vi"("error in (no error)"=w1204, "graph_utilities in"=w1205) -> ("error out"=w1212:errorcluster, "XY Graph"=w1211:refnum<vi>)  [unwired: 6 in, 2 out]
            n505 = Build Path(base path=w1201, name or relative path=w1209) -> (appended path=w1197:path)
            n506 = call <userlib>:"XY Graph to Igor Graph.vi"("error in (no error)"=w1212, "XY Graph Reference"=w1211, "Path"=w1197) -> ("error out"=w1210:errorcluster)  [unwired: 7 in, 1 out]
          }
          frame "V Cut 1" {
            n507 = local read "Intensity 1"() -> (w1214:T7)
            n508 = Unbundle By Name(w1230) -> ("V 1"=w1223:refnum<class "graph_utilities.lvclass">)
            n509 = call <userlib>:"Get Intensity Graph Cursor (Control).vi"("error in (no error)"=w1222, "graph_utilities in"=w1223) -> ("error out"=w1220:errorcluster, "Cursor.Cursor Position"=w1224:T20, "graph_utilities out"=w1221:refnum<class "graph_utilities.lvclass">)  [unwired: 7 in]
            n510 = Unbundle By Name(w1224) -> ("X"=w1216:dbl)
            n511 = Format Into String(format string="%s-%s-%s-%f-", w1217, w1214, w1215, w1216) -> (resulting string=w1226:string)  [unwired: 2 in, 1 out]
            n512 = call <userlib>:"Read XY Graph ref.vi"("error in (no error)"=w1220, "graph_utilities in"=w1221) -> ("error out"=w1229:errorcluster, "XY Graph"=w1228:refnum<vi>)  [unwired: 6 in, 2 out]
            n513 = Build Path(base path=w1218, name or relative path=w1226) -> (appended path=w1219:path)
            n514 = call <userlib>:"XY Graph to Igor Graph.vi"("error in (no error)"=w1229, "XY Graph Reference"=w1228, "Path"=w1219) -> ("error out"=w1227:errorcluster)  [unwired: 7 in, 1 out]
          }
          frame "Intensity 2" {
            n515 = local read "Intensity 2"() -> (w1235:T7)
            n516 = Format Into String(format string="%s-%s-%s-", w1234, w1235, w1231) -> (resulting string=w1237:string)  [unwired: 2 in, 1 out]
            n517 = Unbundle By Name(w1243) -> ("Intensity 2"=w1240:refnum<class "graph_utilities.lvclass">)
            n518 = Build Path(base path=w1233, name or relative path=w1237) -> (appended path=w1232:path)
            n519 = call <userlib>:"Read Intensity Graph ref.vi"("error in (no error)"=w1239, "graph_utilities in"=w1240) -> ("error out"=w1241:errorcluster, "Intensity Graph"=w1242:refnum<vi>)  [unwired: 6 in, 2 out]
            n520 = call <userlib>:"Intensity Graph to Igor Graph.vi"("error in (no error)"=w1241, "Intensity Graph Reference"=w1242, "Path"=w1232) -> ("error out"=w1238:errorcluster)  [unwired: 7 in, 1 out]
          }
          frame "H Cut 2" {
            n521 = local read "Intensity 2"() -> (w1251:T7)
            n522 = Unbundle By Name(w1260) -> ("H 2"=w1248:refnum<class "graph_utilities.lvclass">)
            n523 = call <userlib>:"Get Intensity Graph Cursor (Control).vi"("error in (no error)"=w1246, "graph_utilities in"=w1248) -> ("error out"=w1245:errorcluster, "Cursor.Cursor Position"=w1249:T20, "graph_utilities out"=w1247:refnum<class "graph_utilities.lvclass">)  [unwired: 7 in]
            n524 = Unbundle By Name(w1249) -> ("Y"=w1244:dbl)
            n525 = Format Into String(format string="%s-%s-%s-%f-", w1252, w1251, w1250, w1244) -> (resulting string=w1255:string)  [unwired: 2 in, 1 out]
            n526 = call <userlib>:"Read XY Graph ref.vi"("error in (no error)"=w1245, "graph_utilities in"=w1247) -> ("error out"=w1259:errorcluster, "XY Graph"=w1258:refnum<vi>)  [unwired: 6 in, 2 out]
            n527 = Build Path(base path=w1256, name or relative path=w1255) -> (appended path=w1253:path)
            n528 = call <userlib>:"XY Graph to Igor Graph.vi"("error in (no error)"=w1259, "XY Graph Reference"=w1258, "Path"=w1253) -> ("error out"=w1257:errorcluster)  [unwired: 7 in, 1 out]
          }
          frame "V Cut 2" {
            n529 = local read "Intensity 2"() -> (w1270:T7)
            n530 = Unbundle By Name(w1277) -> ("V 2"=w1265:refnum<class "graph_utilities.lvclass">)
            n531 = call <userlib>:"Get Intensity Graph Cursor (Control).vi"("error in (no error)"=w1262, "graph_utilities in"=w1265) -> ("error out"=w1263:errorcluster, "Cursor.Cursor Position"=w1266:T20, "graph_utilities out"=w1264:refnum<class "graph_utilities.lvclass">)  [unwired: 7 in]
            n532 = Unbundle By Name(w1266) -> ("X"=w1261:dbl)
            n533 = Format Into String(format string="%s-%s-%s-%f-", w1271, w1270, w1269, w1261) -> (resulting string=w1273:string)  [unwired: 2 in, 1 out]
            n534 = call <userlib>:"Read XY Graph ref.vi"("error in (no error)"=w1263, "graph_utilities in"=w1264) -> ("error out"=w1276:errorcluster, "XY Graph"=w1275:refnum<vi>)  [unwired: 6 in, 2 out]
            n535 = Build Path(base path=w1268, name or relative path=w1273) -> (appended path=w1267:path)
            n536 = call <userlib>:"XY Graph to Igor Graph.vi"("error in (no error)"=w1276, "XY Graph Reference"=w1275, "Path"=w1267) -> ("error out"=w1274:errorcluster)  [unwired: 7 in, 1 out]
          }
        }
        n537 = call <vilib>:"Add State(s) to Queue__jki_lib_state_machine.vi"("State(s) in (\"\")"=w1183) -> ("States Out"=w1182:string)  [unwired: 14 in]
      }
    }
  }
  n538 = disable-structure shown="Enabled" {
    frame Disabled {
      n539 = call "Transconductance state machine.vi"() -> ()  [unwired: 12 in]
      n540 = call <userlib>:"TDMS Read Example.vi"() -> ()  [unwired: 12 in]
    }
    frame Enabled {
    }
  }
